vi "Argos_3.5 (K5 Customized Edition).vi"(0 "PID 1 COM":refnum<visa-resource-name>="COM1", 1 "START":bool, 2 "Write to File":bool, 3 "SP 1 input (°C)":dbl=20.0 min=0.0 max=1300.0, 4 "Intervall (s)":u32 max=600, 5 "Write/\nRead":bool=TRUE, 6 "Delay (ms)":u32=500 min=100 max=600000, 7 "Auto Tune":bool, 9 "Standby":bool, 11 "Reset\nSTOPP":bool, 12 "ON":bool=TRUE caption="OFF", 13 "Get Values":bool, 15 "File Path":path) -> (8 "(°C)":dbl format="%#.3f", 14 "SP 1 is (°C)":dbl)   [LabVIEW 2013]
doc: "1. Verwendung\n\nDas Programm dient der Steuerung und Abfrage des Thermocontrollers I3252 und dem Auslesen von zwei VC 840 Messgeräten und einem Druckmessgerät Pfeiffer Single Gauge. \nDie Messgeräte werden Standardmäßig ausgelesen und erst nach Betätigung des Schalters \"Write to File\" in einer Textdatei abgespeichert. Das Eingabefeld \"Intervall\" legt den Abstand der Messpunkte fest.\nDer Setpoint für den Thermocontroller wird erst nach Betätigung des Tasters \"Setpoint START\" übernommen und angesteuert. Er wird ind den EEPROM des Gerätes geschrieben. Die Regelung kann mit Hilfe des Schalters \"Standby\" unterbrochen werden. Durch den Taster \"Reset STOPP\" kann der Setpoint aus dem EEPROM gelöscht werden.\nDie Eingabeflächen \"Constant\" und \"Thickness\" dienen der Berechnung des spezifischen Widerstands.\nDie Eingabeflächen \"User\" und \"Sample\" werden in den Header der Textdatei übernommen.\nDer Indikator \"File Path\" zeigt den aktuellen Speicherort der Textdatei an. Dieser wird nach ausschalten des Schalters \"Write to File\" gelöscht. Bei erneuten Schreiben muss ein neuer Speicherort gewählt werden. Bei Wahl desselben Speicherorts werden sämtliche bereits gespeicherte Daten gelöscht.\n\n\n2. Erläuterungen zum Blockdiagramm\n2.1 äußere Sequenz\nDie äußerte Sequenz besteht aus fünf Frames. Der erste dient der Initialisierung der Ports. Der zweite dient als Verzögerung um dem Programm genug Zeit zu geben die Ports zu öffnen. Jedoch senden die beiden VC 840 bereits Informationen an den Computer die in einem Puffer zwischengespeichert werden. Im dritten Frame wird dieser Puffer geleert. Somit kommt es zu keinem Framing Error. Desweiteren wird in diesem Frame die Startzeit der Messungen genommen. Im vierten Frame wird die eigentliche Messung und Verarbeitung der Daten durchgeführt. Die while-Schleife wird nur durch Auftreten eines Fehlers oder durch Betätigung des Stopbuttons auf dem Front Panel in der oberen linken Ecke unterbrochen. Im fünften und letzten Frame werden die Ports wieder geschlossen und beim Auftreten eines Fehlers wird das Programm automatisch gestoppt. Falls kein Fehler auftritt wird die Sequenz von vorne abgearbeitet.\n\n2.2 while-Schleife und innere Sequenz\n2.2.1 \"Event Structure\"\n2.2.1.1 Allgemein\nDer erste Frame beinhaltet ein \"Event Structure\". Dieser reagiert auf insgesamt elf verschiedene Ereignisse. Falls keines dieser Ereignisse auftreten sollte, warte die Struktur eine Millisekunde bevor die \"Event Structure\" verlassen wird. Die übrigen Ereignisse treten ein, wenn der entsprechende Kontroller eine Werteänderung erfährt.\n\n2.2.1.2 Event: Setpoint\nDieser Case besteht von außen nach innen aus einer Stacked Sequence, einer for-Loop und einer Flat Sequence die wiederum zwei \"Case Structures\" enthält. Als erstes wird bei dem Schalter \"Setpoint START\" der Blinkmodus aktiviert und bei dem Schalter \"Read Temperature\" deaktiviert. Danach folgt das eigentliche setzen des Temperatursollwerts. In der ersten Iteration wird dem Controller I3252 ein Schreibbefehl gesendet. Theoretisch kann der Setpoint in den RAM oder in den EEPROM geschrieben werden. Diese Auswahl erfolgt mit Hilfe des Schalters \"RAM\". Da das Schreiben in den RAM -Speicher aber aus diversen Gründen nicht erwünscht ist, wurde es nicht implementiert. Eine nachträgliche Implementierung ist aber leicht möglich, in dem die untere String-Konstante \"*P012\" durch \"*W012\" ersetzt wird. An diesem Befehl wird eine fünfstellige Hexadezimalzahl angehängt, die den Sollwert wiedergibt. Der Sollwert wird vorher mit zehn multipliziert, da das Komma standardmäßig nach der ersten Ziffer festgesetzt wurde (Bsp.: 800 wird gesendet um 80 einzustellen). Dieser Befehlsstrang wird an das Gerät mittels des SubVIs \"Comm_Interface\", auf welches später noch näher eingegangen wird, weitergegeben. Der durch das Gerät zurückgegebene String wird nicht verarbeitet.\nDie zweite Iteration dient dem Auslesen des eingestellten Sollwertes. Wahlweise kann der RAM- oder der EEPROM-Speicher ausgelesen werden. Die eigentliche Verarbeitung des Ausgabestrings erfolgt durch das SubVI \"Edit Setpoint\".\nDie Implementierung zur Einstellung des zweiten Setpoints erfolgt durch kopieren der ersten beiden Fälle und ersetzen der \"1\" im Befehf durch eine \"2\" (Bsp.: \"*P012\" zu \"*P022\"). Es darf aber nicht vergessen werden, dass dann ebenfalls die Anzahl der Iterationen angepasst werden muss.\nAls letztes wird der Blinkmodus des Schalters \"Setpoint START\" wieder deaktiviert.\n\n2.2.1.3 Event: Standby\nDieses Ereignis aktiviert bzw. deaktiviert als erstes den Blinckmodus des entsprechenden Schalters und sendet danach den Befehl zum aktivieren (\"*D03\") oder zum deaktivieren (\"*E03\") des Standbymodus an den Thermocontroller.\n\n2.2.1.4 Event: Set Command \nDer in das Feld \"Command shall be\" eingegebene Befehl wird an den Thermocontroller übermittlet. Die korrekte Form des Befehls ist im \"Communication Manuel\" nachzuschlagen. Das \"*\"-Zeichen wurde allerdings schon implementiert und muss somit nicht mit eingegeben werden.\n\n2.2.1.5 Event: Reset\nIn der ersten Iteration wird der Reset-Befehl an den Thermocontroller gesendet. In Folge wird der gesamte EEPROM-Speicher gelöscht. Deshalb wird in der zweiten Iteration der Setpoint aktualisiert. Dieser Befehl hat keinen Einfluss auf den RAM-Speicher. Die anschließende Wartezeit ist auf vier Sekunden festgesetzt und wurde empirisch ermittelt. Diese Zeit benötigt das Gerät um den Reset durchzuführen und für die Kommunikation wieder zur Verfügung zu stehen.\n\n2.2.1.6 Event: Auto Tune\nEs ist festgeschrieben, dass der Setpoint für die \"Auto Tune\"-Funktion wenigstens 20°C über der aktuellen Temperatur liegt. Deshalb wird zunächst der aktuelle Temperaturwert ausgelesen. Im zweiten Schritt werden zu diesem Wert zwanzig addiert und der Setpoint wird in den RAM-Speicher geschrieben. Das Schreiben in diesen Speicher ist nötig, da die \"Auto Tune\"-Funktion\" erst nach einem Reset startet. Im dritten Schritt wird der eigentliche Befehl für den \"Auto Tune\" gesendet (siehe dazu \"Communication Manuel\" S.27). Als vierte und letzte Iteration der for-Schleife folgt der bereits erwähnte Reset-Befehl. Der Temperatursollwert, der im RAM-Speicher eingetragen ist, muss zum Schluss wieder auf 0°C gesetzt werden. Die Zeit für die Ausführung des \"Auto Tune\"-Befehls wurde empirisch ermittelt und 45 s festgesetzt.\n\n2.2.1.7 Event: Write LOW/HI\nDieses Ereignis setzt die am Analogausgang anliegende Spannung fest. Normalerweise beträgt dieser Spannungswert 0-10 V. Das angeschlossene Netzteil verträgt aber maximal nur 2,3 V. Aus diesem Grund wird der \"%HIGH\" auf 23 gesetzt. Somit beträgt die maximal anliegende Spannung nur noch 23% von der maximal möglichen, d.h 2,3V. Ein niedrigerer Wert ist jederzeit möglich, genauso wie ein höherer für den Parameter \"%LOW\". Diese werden zunächst nacheinander in den RAM-Speicher geschrieben und anschließend wieder ausgelesen.\n\n2.2.1.8 Event: Set PID\nDie Werte für den PID-Regler können sowohl mit Hilfe der \"Auto Tune\"-Funktion, als auch manuell eingestellt werden. Es wird wiederum zwischen dem Schreiben in den RAM- und dem EEPROM-Speicher unterschieden. Zunächst werden die Werte für \"P\", \"I\" und \"D\", in dieser Reihenfolge, gesetzt und danach die aktuellen Werte ausgelesen.\n\n2.2.1.9 Event: Get Values\nDieses Ereignis hat zur Folge, dass die Werte für \"P\", \"I\", \"D\", \"%LOW\", \"%HIGH\" und des Setpoints wahlweise aus dem RAM- oder EEPROM-Speicher gelesen werden. Die aktuellen Werte werden nicht nur in die entsprechenden Anzeigefelder übernommen, sondern auch in die entsprechenden Eingabefelder, mit Ausnahme des Temperatursollwerts. \n\n2.2.1.10 Event: RAM\nPrinzipiell kann zwischen dem Schreiben in den RAM- oder EEPROM-Speicher des Thermocontrollers gewählt werden. Die entsprechende Schalterposition auf dem Frontpanel zeigt den aktuell verwendeten Speicher an. Die Anzeigewerte werden bei jedem Umschalten aktualisiert und sind im entsprechenden Speicher eingetragen. Die Implementierung ist identisch mit der des Ereignisses \"Get Values\". Es gilt zu beachten, dass die Werte für \"%LOW\" und \"%HIGH\" nur in den RAM-Speicher geschrieben werden können und somit auch nur aus diesem ausgelesen werden können.\n\n2.2.1.11 Event: Set Gauge to Zero\nMit Hilfe der SubVIs \"Get Pressure\" und \"Offset Display\" werden die Werte für den alten und den neuen Offset und der durch den zweiten Drucksensor ermittelt Druck ermittelt. \n\n2.2.1.12 Event: Write to File\nSollte der Schalter \"Write to File\" aktiviert werden, d.h. Schalterposition oben, so wird zunächst durch das SubVI \"Header\" ein Header für die unter \"File Path\" definierte Datei angelegt. Alle Werte, die bereits in der entsprechenden Datei stehen, werden dabei gelöscht.\n\n2.2.2 \"Timed Structures\"\nIm dritten Frame der inneren Sequenz werden die Werte für Zeitpunkt, Temperatur, Spannung, Strom und Druck ermittelt. Damit die Werte zum gleichen Zeitpunkt aufgenommen werden, werden \"Timed Sequences\" eingesetzt. Mit dem entsprechenden Schalter auf dem Front Panel unter dem Tab \"Settings\" kann gewählt werden, ob das entsprechende Gerät ausgelesen werden soll oder nicht. Die einzelnen Sequenzen werden parallel abgearbeitet, womit die Prozesszeit von diesem Frame durch der zeitintensivsten Sequenz abhängt. Dies ist in aller Regel das Auslesen der Temperatur, da ein \"Delay\" von 500 ms oder größer benötigt wird, um den Controller ordentlich ansprechen zu können.\nDie Systemzeit wird durch das SubVI \"System Time in Seconds\" in Sekunden umgerechnet und der in dem Parameter \"Starttime\" gespeicherte Wert wird abgezogen. Somit werden die Sekunden seit dem Start des Programms gezählt.\n\n2.2.3 restlichen Frames\nIm zweiten Frame wird das Intervall zwischen den einzelnen Messwerten festgelegt. Dabei wird der Wert des Parameters \"Delay\" abgezogen. Dieser Wert beträgt im Normalfall 500 ms und ist somit nicht vernachlääsigbar.\nDer Vierte Frame beinhaltet die Umrechnung des Temperatur-Strings in einen Temperaturwert durch das SubVI \"Edit Tmperature\", die Berechnung des spezifischen Widerstands durch das SubVI \"Resistivity Calculation\" und die Überprüfung des Druckwerts. Auch werden die neu gewonnen Werte in das entsprechende Shift-Register übernommen. Falls der Druckwert einen in dem Parameter \"Pressure Limit (mbar)\" festgelegten Grenzwert überschreiten sollte, wird der Thermocontroller automatisch in den Standby-Modus versetzt. Des Weiteren wird der Schalter \"Standby\" solange gesperrt, wie der Druck oberhalb des Grenzwertes liegt. Wenn der Druck wieder unter den Grenzwert gesunken ist, wird der Standby-Befehl nicht automatisch aufgehoben, sondern muss vom Benutzer durch Betätigung des entsprechenden Schalters gegeben werden.\nIm fünften Frame werden die Diagramme erstellt. Dabei wird jedes Mal von neuem das gesamte Shift-Register als Graph dargestellt. Weiterhin werden die Messwerte in ein 1D-Array geschrieben.\nDer sechste und letzte Frame beinhaltet den eigentlich Schreibvorgang der Messwerte in eine Textdatei und die Überprüfung ob ein Fehler vorliegt.\n\n2.3 SubVIs\n2.3.1 Allgemein\nDie SubVIs für die Messgeräte VC840 und das Druckmessgerät wurden aus anderen Quellen übernommen. \n\n2.3.2 \"Header\"\nIn den Header wird zunächst das aktuelle Datum und die aktuelle Zeit übernommen. Die ausgewählte Datei wird dabei überschrieben. Danach wird der Name des Benutzers und der Probe übernommen. Zum Schluss werden die Einheiten in einer Reihe, durch einen Tabulator getrennt, in den Header geschrieben.\n\n2.3.3 \"I3252 Comm Interface\"\nDieses VI stellt die Kommunikation mit dem Thermocontroller her und gibt den Ausgabe-String zurück.\n\n2.3.4 \"I3252 Edit Setpoint\"\nIm Ausgabe-String vom Thermocontroller ist an der vierten Stelle die Stelle des Dezimalpunktes verschlüsselt. Dieses Hexadezimalzahl wird herausgefiltert und an ein \"ENUM Controller\" übergeben. Dieser weist der Hexadezimalzahl eine Nummer zu, mit welcher ein Wert aus einem Array entnommen wird. Dieser Wert dient als Quotient. Der tatsächliche Wert kann somit errechnet werden.\n\n2.3.5 \"I3252 Edit Temperature\"\nDer Temperatur-String, der vom Thermocontroller zurückgegeben wird, wird in eine Dezimalzahl umgewandelt. Manchmal kommt es aus zu Dropouts, die durch dieses Programm herausgefiltert werden. Der letzte Wert wird dabei in einer \"Feedback Node\" gehalten unter der Annahme, dass sich der Temperaturwert nicht sprunghaft ändert.\n\n2.3.6 \"Resistivity Calculation\"\nDer spezifische Widerstand wird nach folgender Formel ausgerechnet. Dabei entspricht t der Dicke der Probe und C ist eine Konstante.\nrho=C*pi*t*U/(ln( 2)*I)\n\n2.3.7 \"System Time in Seconds\"\nZunächst wird die aktuelle Systemzeit ausgelesen. Danach wird diese in Stunden, Minuten und Sekunden aufgeteilt, alles in Sekunden umgerechnet und letztendlich addiert."
uses:
  <vilib>/Platform/TimedLoop/XDataNode/timing_clust.ctl
  <vilib>/Platform/TimedLoop/XDataNode/nitl_modes.ctl
  <vilib>/Platform/TimedLoop/XDataNode/wakeup.ctl
  <vilib>/Instr/_visa.llb/VISA Configure Serial Port (Instr).vi
  <vilib>/Platform/TimedLoop/scheduler/LVUserAPI/_suppVIs/Create_1kHz_TSource.vi
  <vilib>/Utility/file.llb/Write To Spreadsheet File (DBL).vi
  <vilib>/Platform/TimedLoop/XDataNode/XDataNode.xnode
  <vilib>/Platform/TimedLoop/XDataNode/XDNodeRunTimeDep.lvlib
  D:/Argos_K_1.99 (SUPTNIK Customized Edition)/Dependencies/Pfeiffer TPG261+262 Single+Dual Gauge/Dual Gauge.lvlib
panel:
  out "Resistivity/ Temp Dependency":cluster{dbl[], dbl[]}(graph)
  out "read buffer":string
  out "appended array":dbl[](array[numeric])
  in  "Tab Control":T1(tab)
  in  "Soak time (min)":dbl
  in  "Ramp time (min)":dbl
  in  "RAMP":bool
  in  "Set Value":bool
  in  "OUTPUT":bool
  in  "4PP Const":dbl=1.0
  in  "Thickness":dbl=40.0
  in  "Voltage\nCompl.":dbl=2.0
  in  "Unit   2":string(combo)="0"
  in  "Unit":string(combo)="1"
  in  "Source \nCurrent":dbl=20.0
  in  "Sample":string
  in  "User":string
  out "Thermocouple":cluster{dbl[], dbl[]}(graph)
  out "current time (s)":dbl
  out "data logger intervall (s)":dbl
  out "loop time (s)":dbl
  in  "stop":bool
  out "TPG 1":cluster{dbl[], dbl[]}(graph)
  out "Pressure Baratron 2":dbl format="%#_4e"
  out "Resistivity Graph":cluster{dbl[], dbl[]}(graph)
  out "Resistivity\n 2":dbl
  out "Voltage Graph":cluster{dbl[], dbl[]}(graph)
  out "Current Graph":cluster{dbl[], dbl[]}(graph)
  out "Voltage\n 2":string
  out "Current \n3":string
  in  "Keithley Port":refnum<visa-resource-name>="COM6"
  out "status 2":bool caption="Status"
  out "code 2":i32 caption="Code"
  out "code":i32 caption="Code"
  out "status":bool caption="Status"
  in  "Set Gauge to Zero":bool
  out "Status Gauge 1#2":i32(ring) items=["data OK", "underrange", "overrange", "sensor error", "sensor off", "no sensor", "ID error"]
  out "Pressure Gauge 1#2":dbl format="%.3e"
  out "Pressure Gauge 1#1":dbl format="%.3e"
  out "Status Gauge 1#1":i32(ring) items=["data OK", "underrange", "overrange", "sensor error", "sensor off", "no sensor", "ID error"]
  in  "TPG 1 COM":refnum<visa-resource-name>="COM5"
  in  "Pressure Limit (mbar)":dbl=1.0 min=0.0 max=1100.0
  out "Current Offset (mbar)":dbl
  in  "ON (TPG 2)":bool caption="OFF"
  in  "ON (TPG 1)":bool=TRUE caption="OFF"
  in  "ON":bool caption="OFF"
  in  "VC 840 2":refnum<visa-resource-name>="COM4"
  out "Reading 2":dbl format="%_4f"
  out "Mode 2":enum16{"?", "Diode", "Beep", "DC", "AC"}(ring)
  out "Unit 2":string
  in  "VC 840 1":refnum<visa-resource-name>="COM4"
  out "Reading 1":dbl format="%_4f"
  out "Mode 1":enum16{"?", "Diode", "Beep", "DC", "AC"}(ring)
  out "Unit 1":string
  out "Status 1":T2
  out "Status 2":T2
  in  "ON":bool caption="OFF"
  out "% HIGH Istwert":u32
  out "% LOW Istwert":u32
  in  "% High Sollwert":u32=23 max=24
  in  "% LOW Sollwert":u32 max=25
  in  "RAM":bool=TRUE caption="EEPROM"
  out "D (Rate) IstWert":u32
  out "I ( Reset1) Istwert":u32
  out "P (PB1) Istwert":u32 caption="actual value"
  in  "D (Rate) Sollwert":u32 max=3999
  in  "I ( Reset1) Sollwert":u32 max=3999
  in  "P (PB1) Sollwert":u32 caption="set value" max=9999
  in  "Set Command":bool
  in  "Set PID":bool
  in  "Write LOW/HI":bool
  in  "Flow Control":u16(ring) items=["None"=0, "XON/XOFF"=1, "RTS/CTS"=2, "DTR/DSR"=4]
  in  "Stop Bits":u16(ring)=10 items=["1.0"=10, "1.5"=15, "2.0"=20]
  in  "Parity":u16(ring)=1 items=["None", "Odd", "Even", "Mark", "Space"]
  in  "Data Bits":u16=7 min=5 max=8 step=1
  in  "Baud Rate":u32=9600
  out "Command output":string
  in  "Command input":string
  in  "TPG 2 COM":refnum<visa-resource-name>="COM4"
  out "Pressure Gauge 2#2":dbl format="%.3e"
  out "Pressure Gauge 2#1":dbl format="%.3e"
  out "Status Gauge 2#2":i32(ring) items=["data OK", "underrange", "overrange", "sensor error", "sensor off", "no sensor", "ID error"]
  out "Status Gauge 2#1":i32(ring) items=["data OK", "underrange", "overrange", "sensor error", "sensor off", "no sensor", "ID error"]
  out "Pirani (VVP1 Scroll)":cluster{dbl[], dbl[]}(graph)
  in  "4PP constant":dbl min=0.0 max=5.0
  in  "Thickness (nm)":dbl min=0.0
  out "Pressure Pirani 2":dbl format="%#_3e"
  in  "Minutes":dbl
  in  "Hours":dbl
  in  "Soak Minutes":dbl=1.0
  in  "Soak Hours":dbl
  out "Actual SetPoint":dbl
  in  "Get SetPoint":bool
  # "set \nvalue"
  # "actual \nvalue"
  # "T (°C)"
  # "nm"
  # "Ohm Cm"
  # "mbar"
  # "Amps"
  # "Pressure Measurement \n(Pfeiffer TPG261)"
  # "PID Controller (Omega Newport i3252)"
  # "Keithley 4PP measurement"
  # "Ramp And Soak Toolkit"
  # "limit (mbar)"
  # "Multimeter\n#1 (VC 840)"
  # "Multimeter\n#2 (VC 840)"
  # "P"
  # "I"
  # "D"
  # "% Low"
  # "% High"
  # "mbar"
  # "Ramp"
  # "Soak"
  # "Authors:  Daniel Schuster (sir-dan@web.de)\n                 Steffen Cornelius (s.cornelius@hzdr.de)\n                 Nico Spahn (x)\n\n                 premade SubVIs for readout of Pfeiffer gauge and VC840 Multimeters were used\n                 SubVI \"I3252_Comm_Interface\" is based on a modified Labview example\n\nRelease:  v1.0    \n\nVersion History:\n\nv1.1  -    28.06.2011\n             - Format des Files geändert von %.3f auf %g\n             - maximale Eingabewerte für PID begrenzt\nv1.2  -    12.07.2011\n             - Anzeige p,rho, U, V auf Scientific geändert\n             - y-Achse p,rho auf Log geändert\n             - numerische Zeitanzeige hinzugefügt\n             - 4PP Constant: pi/ln(2)=4,532 set as the default value\nv1.3  -    25.07.2011\n             - Zeitvariable auf EXT geändert, um Sprünge in Diagrammen loszuwerden\nv1.4  -   27.07.2011\n             - ALLE Variablen auf DBL zurückgesetzt wegen Formatierungsproblem im File\n             - Zeitberechnung neu gemacht (Tick count differenzen) -> Zeitsprünge korrigiert ?\n             - Delay/Intervall überarbeitet\nv1.5  -   05.12.2012\n                - Austausch der alten Pfeifer SubvIs durch neue -> nun alle 4 Kanäle des DualGauge\n                                                                                                         Controllers gleichzeitig auslesbar\n                - neue Pfeiffer SubVIs verwendet in Druckwertauslesung und Offset Berechnung des Baratron\n                  Druckes (COM5 Sensor1)\n                - Neuarragement des GUI -> FullRange und Baratron neben Temperatur auf Haupseite zu sehen\n                                                                   Pirani und OpenPort auf Meas.2 zu sehen\n                                                                   Diagnose Seite umfasst nun auch Widerstandsdiagramm\n                - Änderungen der Settingseite -> nun alle 4 Drucksensoren mit aktuellem Messwert und Gerätestatus\n                                                                           zu sehen\n                - The readout of the PID-Temperature Controller and the VC840 Multimeters was not modified\nv1.73  -  18.10.2013\n                - Layout Änderungen\nv.1.8   -  19.01.2014\n                - Änderung Layout Settings Tab\n                - Trennung der beiden TPG Dual Gauge Controls\n                -"
  # "Version 1.73    - last change 18.10.2013"
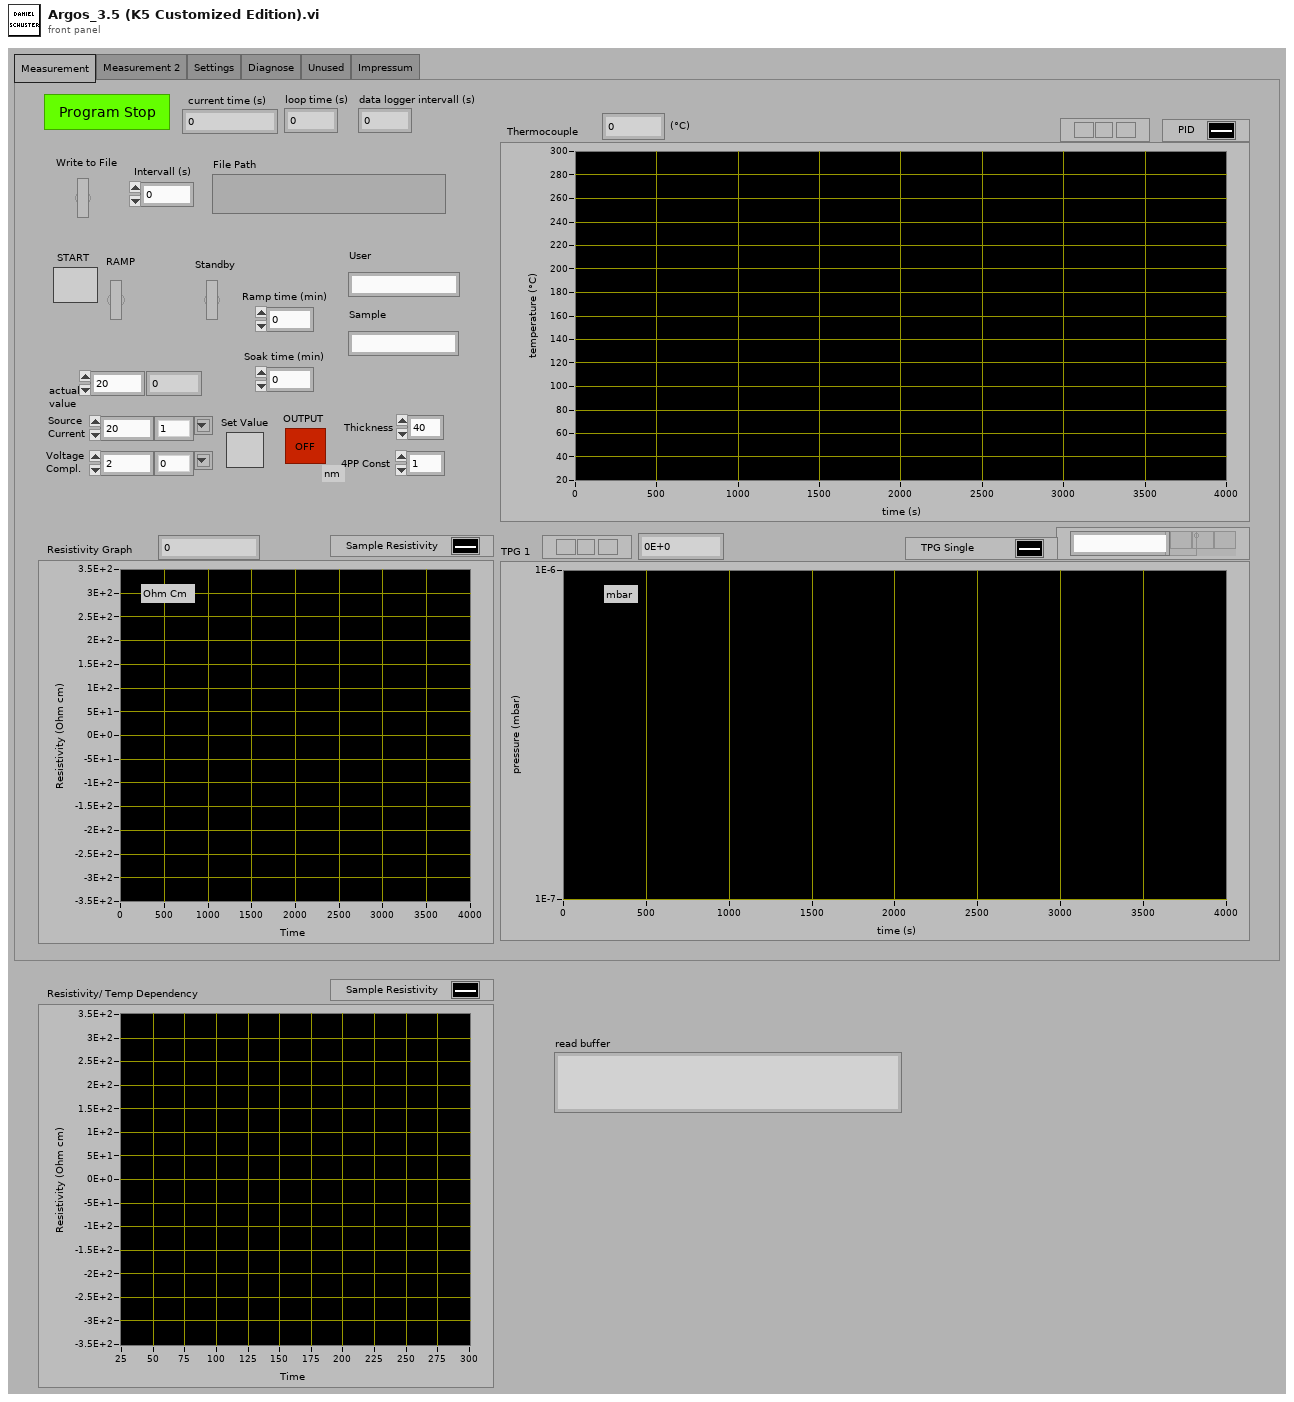
[diagram p1: front panel]
types:
  T1 = enum32{"Measurement", "Measurement 2", "Settings", "Diagnose", "Unused", "Impressum"}
  T2 = cluster{"Low Bat":bool, "Auto":bool, "Delta":bool, "Hold":bool, "RS232":bool}
  T3 = typedef "XDNodeRunTimeDep.lvlib/timing_clust.ctl" = cluster{"Expected End [f-1]":u64, "Actual End [f-1]":u64, "Finished Late? [f-1]":bool, "Expected End [i-1]":u64, "Actual End [i-1]":u64, "Finished Late? [i-1]":bool, "Expected Start [i]":u64, "Actual Start [i]":u64, "Expected Start [f]":u64, "Actual Start [f]":u64, "Source Name":string, "Structure Name":string, "Period":i64, "Deadline":i64, "Offset":i64, "Start":i64, "Priority":i32, "Timeout":i32, "Mode":T4, "Wakeup Reason":T5, "Error":errorcluster, "Source Type":string, "Secondary Source Type":string, "Global End Time":u64, "Global Start Time":u64, "Frame Duration":u64, "Iteration Duration":u64, "Assigned CPU":i32, "I/O Scan Engine Mode":u32}
  T4 = typedef "XDNodeRunTimeDep.lvlib/nitl_modes.ctl" = enum32{"No Change", "Process missed periods, maintain original phase", "Discard missed periods, maintain original phase", "Process missed periods, ignore original phase", "Discard missed periods, ignore original phase"}
  T5 = typedef "XDNodeRunTimeDep.lvlib/wakeup.ctl" = enum32{"Normal", "Aborted", "Asynchronous wakeup", "Timing source error", "Timed loop error", "Timeout"}
  T6 = enum8{"Enabled", "Disabled", "Disabled and Grayed Out"}
  T7 = cluster{"VISA resource name out":refnum<visa-resource-name>, "error out":errorcluster, "Delay (ms)":u32, "Write/\nRead":bool}
  T8 = cluster{"TPG 2 COM":refnum<visa-resource-name>, "error out":errorcluster}
  T9 = cluster{"COM out":refnum<visa-resource-name>, "Cluster (Ausgang)":errorcluster}
  T10 = cluster{"Pressure Gauge#1":dbl, "Pressure Gauge#2":dbl}
  T11 = cluster{"TPG 1 COM":refnum<visa-resource-name>, "error out":errorcluster}
  T12 = cluster{"COM out":refnum<visa-resource-name>, "error out":errorcluster, "COM out":refnum<visa-resource-name>, "error out":errorcluster}
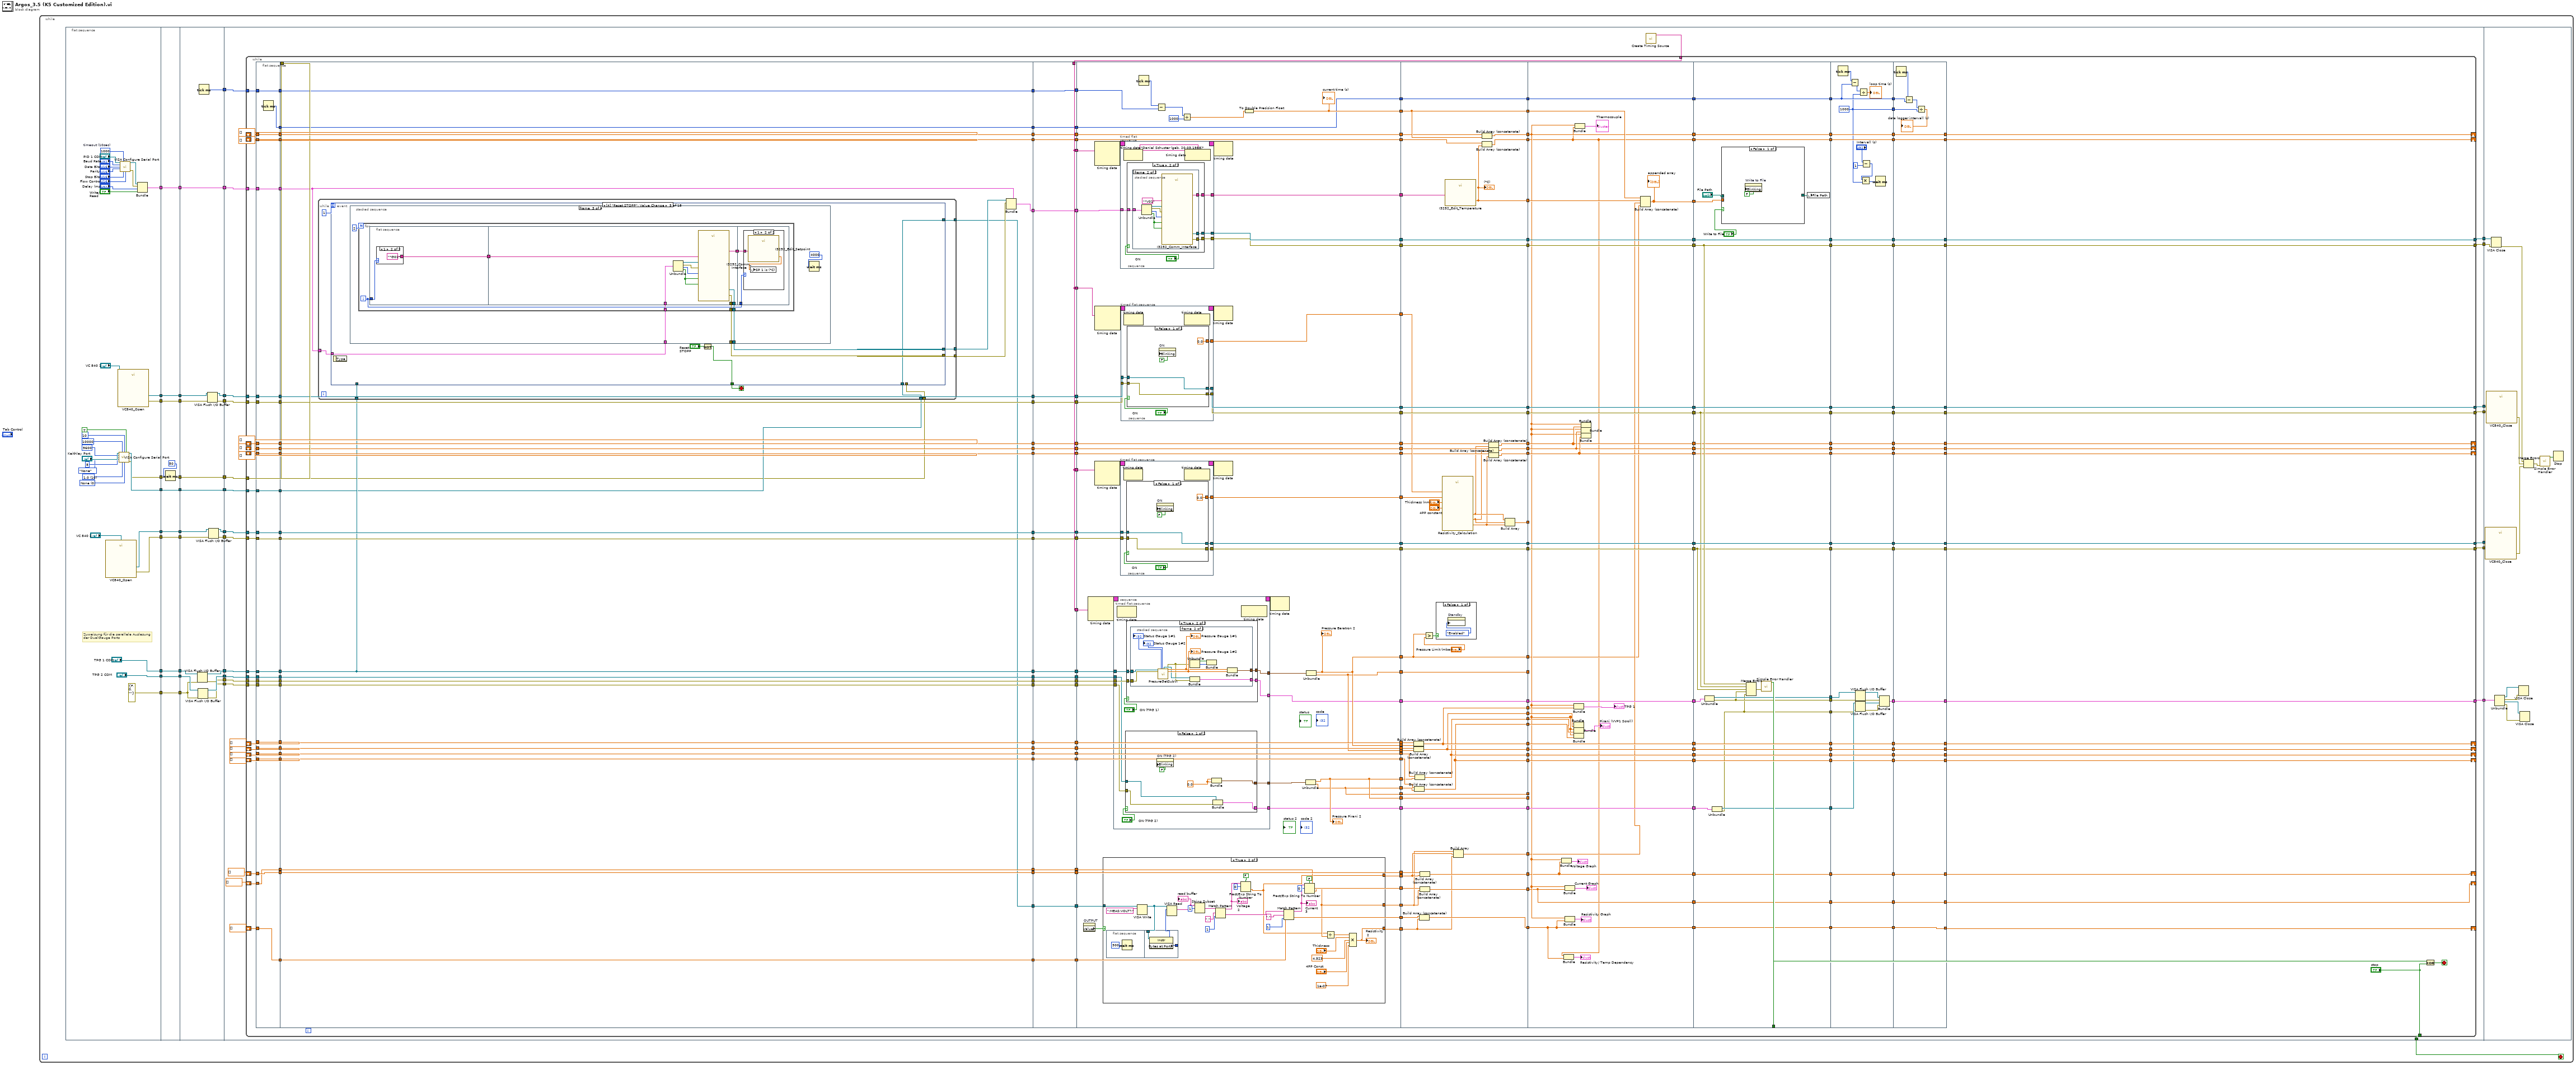
[diagram p0: block diagram]
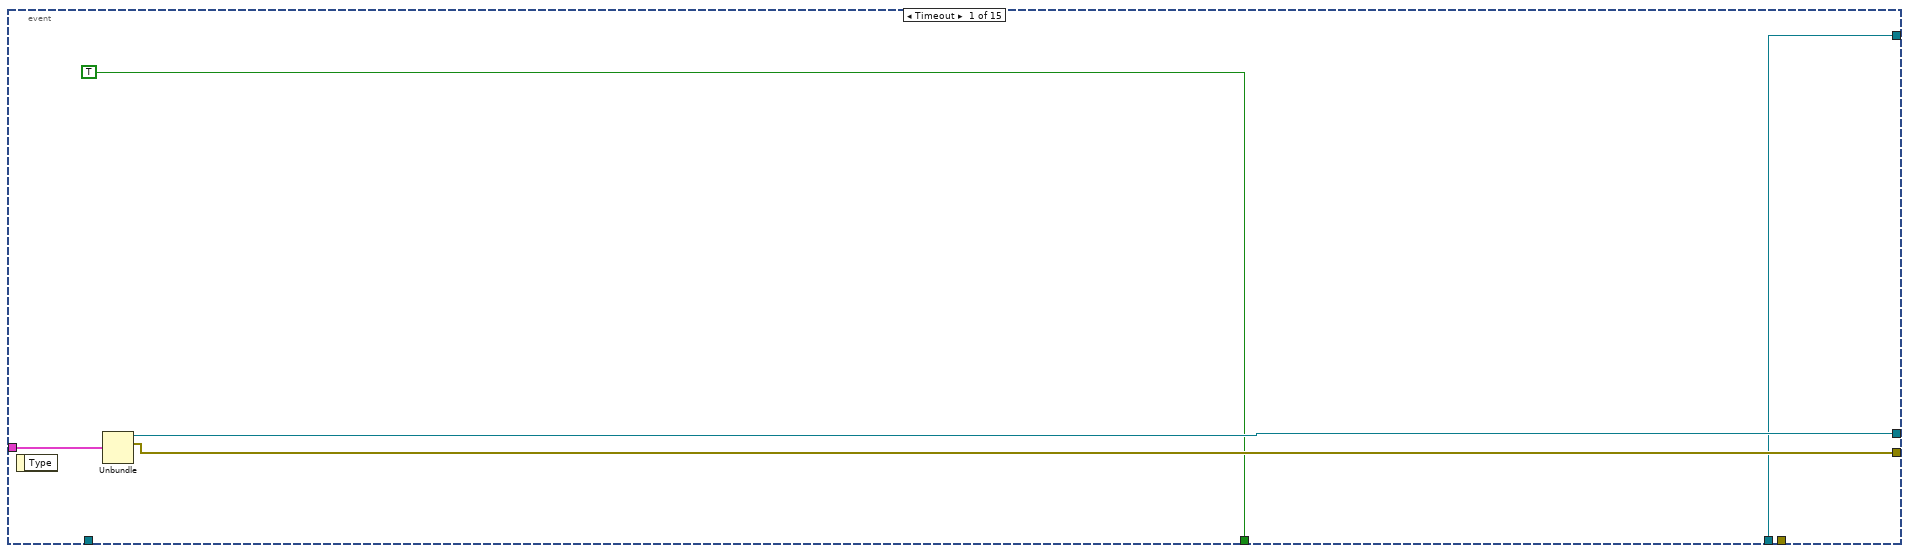
[diagram p2: hidden frame]
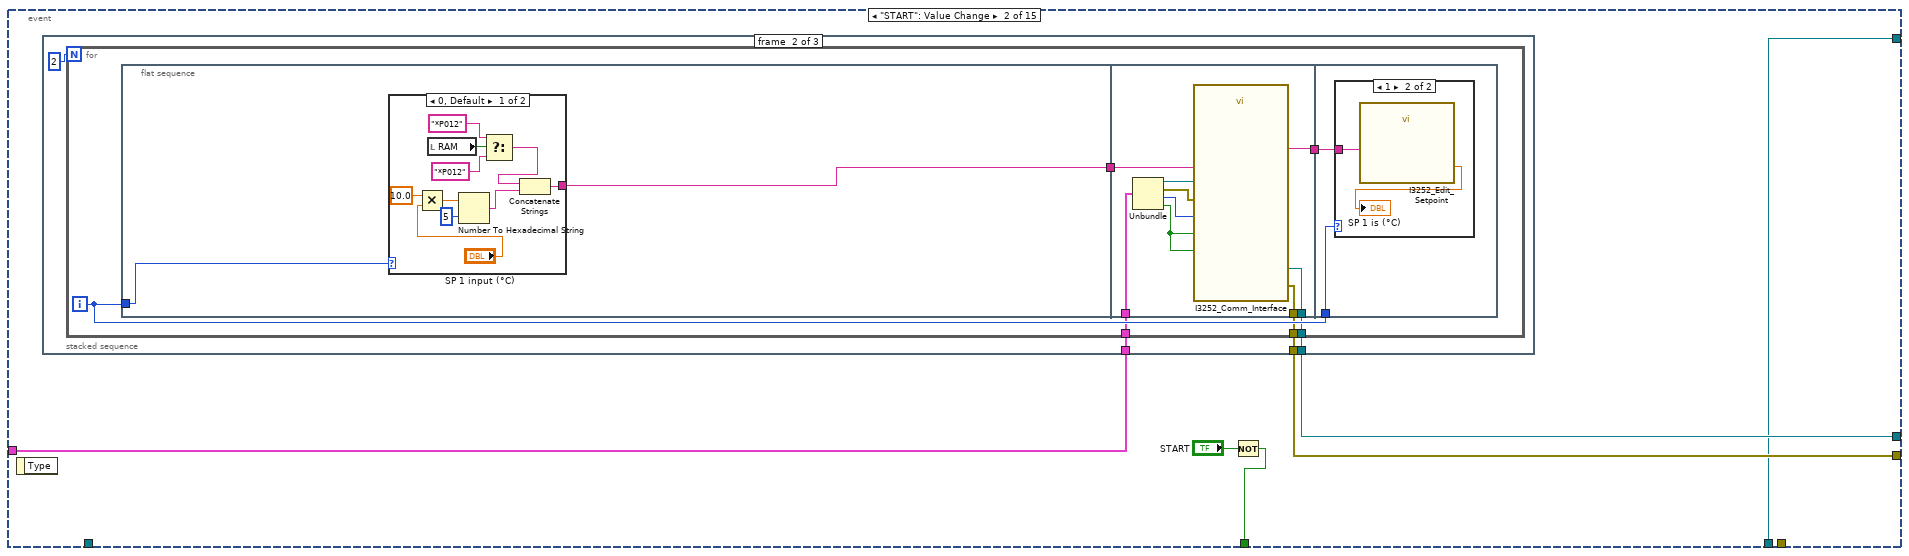
[diagram p3: hidden frame]
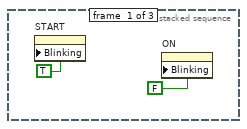
[diagram p4: hidden frame]
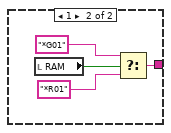
[diagram p5: hidden frame]
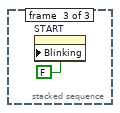
[diagram p7: hidden frame]
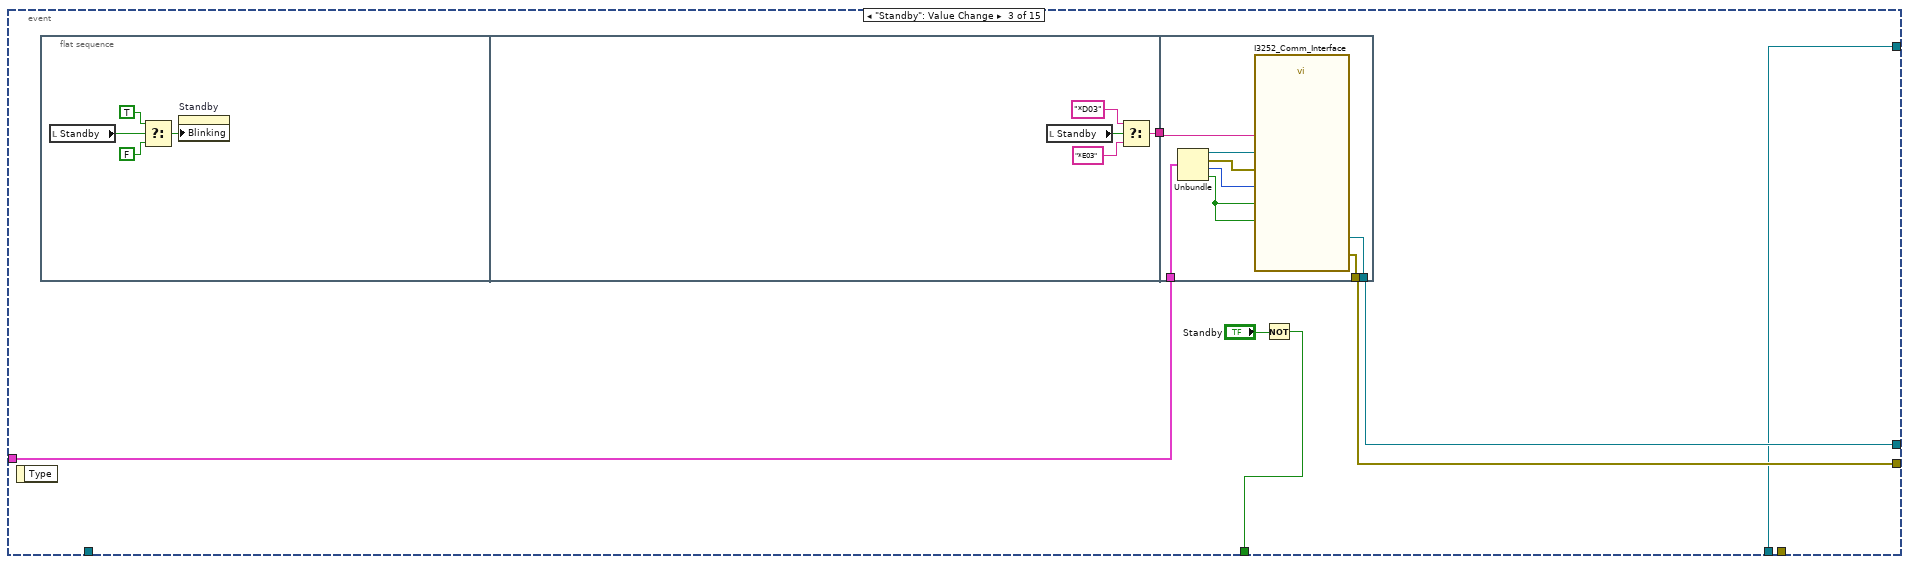
[diagram p8: hidden frame]
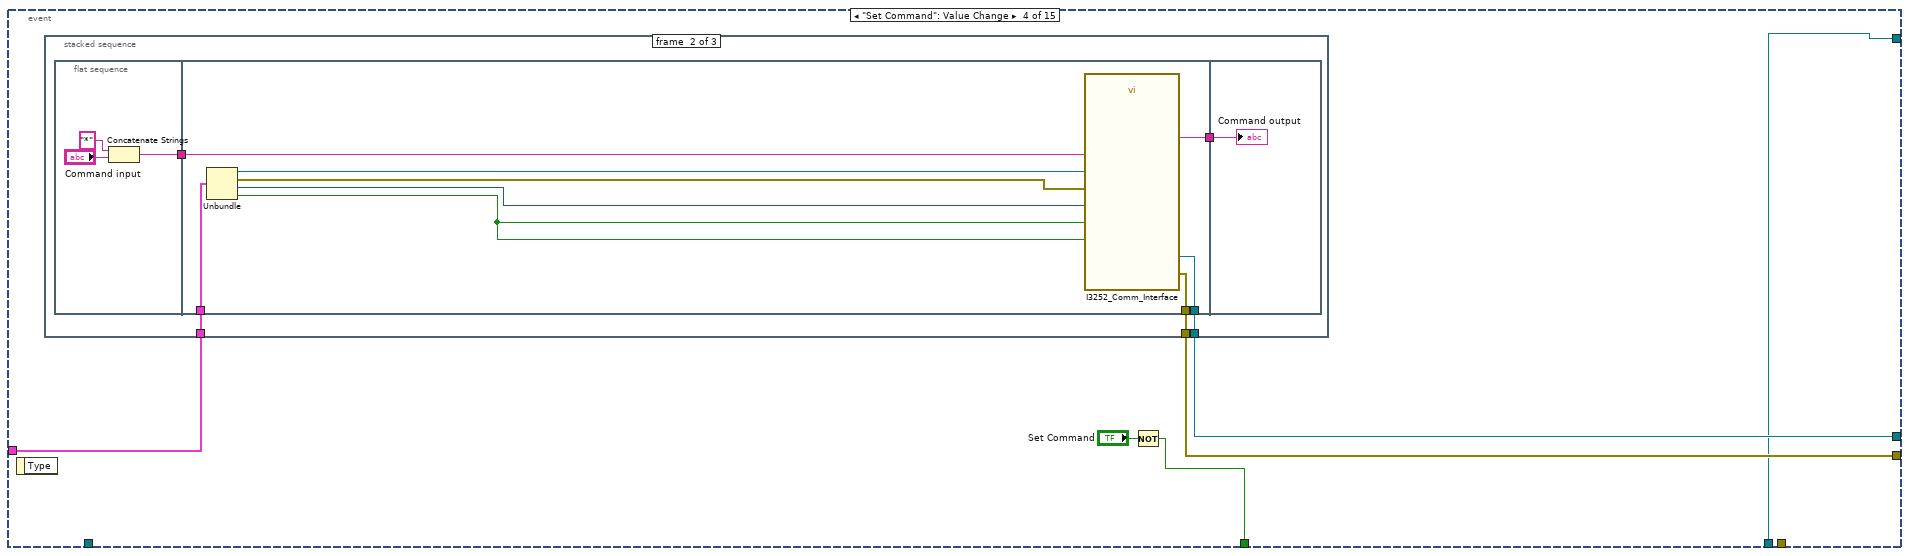
[diagram p9: hidden frame]
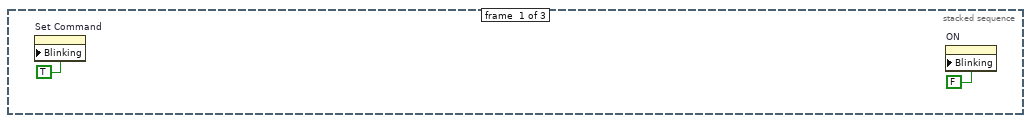
[diagram p10: hidden frame]
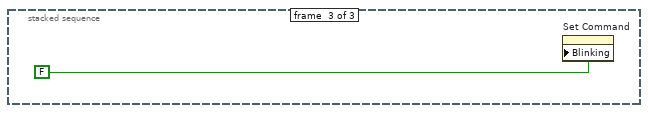
[diagram p11: hidden frame]
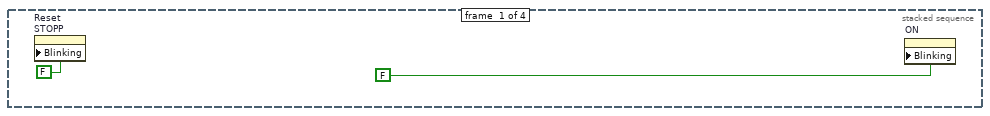
[diagram p12: hidden frame]
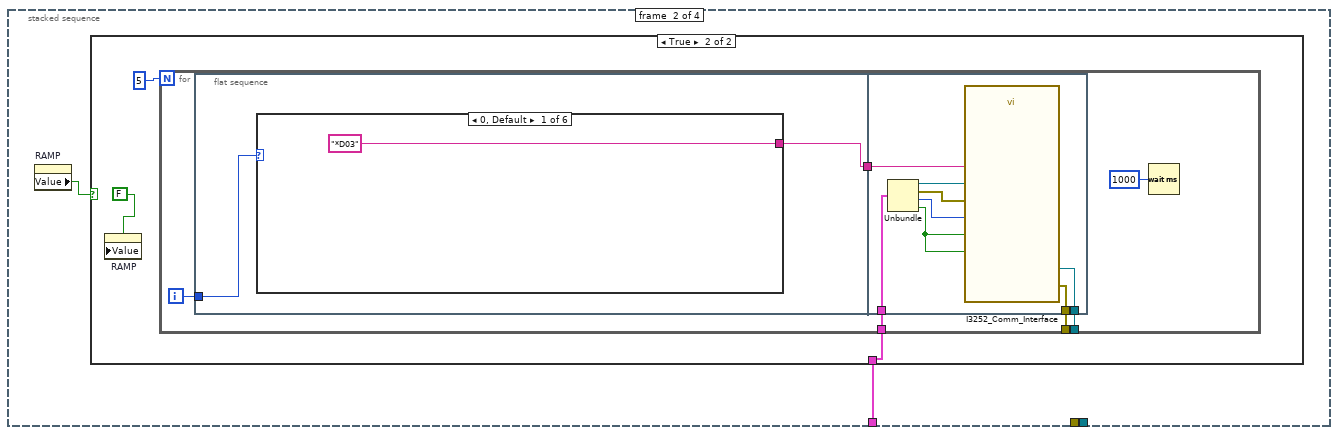
[diagram p13: hidden frame]
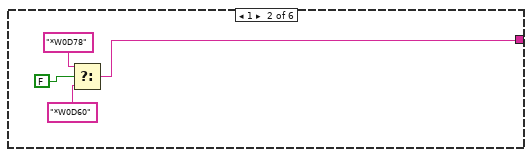
[diagram p15: hidden frame]
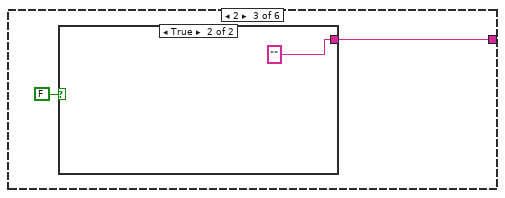
[diagram p16: hidden frame]
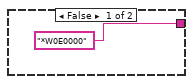
[diagram p17: hidden frame]
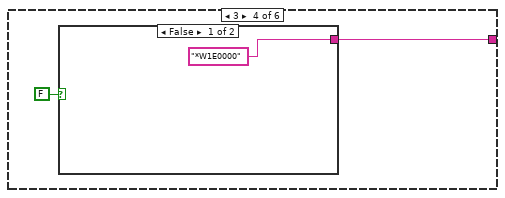
[diagram p18: hidden frame]
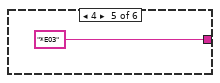
[diagram p20: hidden frame]
diagram:
  n1 = while {
    stop <- w12 stop-if-true
    n2 = flat-sequence {
      tunnel: [w71] -> w40
      tunnel: [w72] -> w39
      tunnel: [w57] -> w38
      tunnel: [w70] -> w37
      tunnel: [w69] -> w36
      tunnel: ["TPG 1 COM"] -> w35
      tunnel: ["TPG 2 COM"] -> w34
      tunnel: [errorcluster {"status"=FALSE, "code"=0, "source"=""} ("Fehler (Eingang)")] -> w9
      tunnel: [w42] -> w4
      tunnel: [w41] -> w3
      tunnel: w40 -> [w83]
      tunnel: [w83] -> w33
      tunnel: w39 -> [w82]
      tunnel: [w82] -> w32
      tunnel: w38 -> [w81]
      tunnel: [w81] -> w31
      tunnel: w37 -> [w80]
      tunnel: [w80] -> w30
      tunnel: w36 -> [w79]
      tunnel: [w79] -> w29
      tunnel: [w77] -> w28
      tunnel: w35 -> [w77]
      tunnel: [w76] -> w27
      tunnel: w34 -> [w76]
      tunnel: [w75] -> w10
      tunnel: w9 -> [w75]
      tunnel: [w74] -> w5
      tunnel: w4 -> [w74]
      tunnel: w3 -> [w73]
      tunnel: [w73] -> w2
      tunnel: w33 -> [w96]
      tunnel: [w95] -> w26
      tunnel: w32 -> [w97]
      tunnel: [w94] -> w25
      tunnel: w31 -> [w102]
      tunnel: [w102] -> w24
      tunnel: w30 -> [w99]
      tunnel: [w100] -> w23
      tunnel: w29 -> [w98]
      tunnel: [w101] -> w22
      tunnel: [w93] -> w21
      tunnel: [w91] -> w20
      tunnel: w28 -> [w92]
      tunnel: [w90] -> w19
      tunnel: w27 -> [w89]
      tunnel: w10 -> [w88]
      tunnel: [w87] -> w8
      tunnel: [w86] -> w7
      tunnel: [w85] -> w6
      tunnel: w5 -> [w85]
      tunnel: w2 -> [w84]
      tunnel: [w84] -> w1
      tunnel: w26 -> [w135]
      tunnel: w25 -> [w134]
      tunnel: w24 -> [w133]
      tunnel: w23 -> [w131]
      tunnel: w22 -> [w130]
      tunnel: [w129] -> w18
      tunnel: [w128] -> w17
      tunnel: [w127] -> w16
      tunnel: [w126] -> w15
      tunnel: [w125] -> w14
      tunnel: [w124] -> w13
      tunnel: w21 -> [w118]
      tunnel: w20 -> [w117]
      tunnel: w19 -> [w116]
      tunnel: [w111] -> w12
      tunnel: [w110] -> w11
      tunnel: w8 -> [w109]
      tunnel: w7 -> [w108]
      tunnel: w6 -> [w107]
      tunnel: w1 -> [w106]
      tunnel: w18 -> [w1640]
      tunnel: w17 -> [w1639]
      tunnel: w16 -> [w1642]
      tunnel: w15 -> [w1641]
      tunnel: w14 -> [w1644]
      tunnel: w13 -> [w1643]
      tunnel: w11 -> [w1637]
      frame #0 {
        w43 = u16 0 items=["None", "XON/XOFF", "RTS/CTS", "XON/XOFF & RTS/CTS", "DTR/DSR", "XON/XOFF & DTR/DSR"] ("flow control (0:none)")
        w44 = u16 10 items=["1.0"=10, "1.5"=15, "2.0"=20] ("stop bits (10: 1 bit)")
        w58 = u32 1000  # timeout (10sec)
        # "Zuweisung für die parallele Auslesung\nder DualGauge Ports"
        n3 = call "VC840_Open.vi"("VISA resource name"="VC 840 2") -> ("error out"=w69:errorcluster, "VISA resource name out"=w70:refnum<visa-resource-name>)  [unwired: 1 in, 8 out]
        n4 = call "VC840_Open.vi"("VISA resource name"="VC 840 1") -> ("error out"=w72:errorcluster, "VISA resource name out"=w71:refnum<visa-resource-name>)  [unwired: 1 in, 8 out]
        n5 = call-poly "VISA Configure Serial Port"("VISA resource name"="Keithley Port", "timeout (10sec)"=u32 10000, "termination char\n(0xA = '\\n' = LF)"=u8 10 ("termination char\n(0xA = '\\n' = LF)"), "Enable Termination\nChar (T)"=TRUE ("Enable Termination\nChar (T)"), "baud rate (9600)"=u32 9600, "data bits (8)"=u16 8, "parity (0:none)"=enum16{"None", "Odd", "Even", "Mark", "Space"}."None", "stop bits (10: 1 bit)"=w44, "flow control (0:none)"=w43) -> ("VISA resource name out"=w42:refnum<visa-resource-name>, "error out"=w41:errorcluster)  [unwired: 5 in]
        n6 = call-poly "VISA Configure Serial Port"("VISA resource name"="PID 1 COM", "timeout (10sec)"=w58, "baud rate (9600)"="Baud Rate", "data bits (8)"="Data Bits", "parity (0:none)"="Parity", "stop bits (10: 1 bit)"="Stop Bits", "flow control (0:none)"="Flow Control") -> ("VISA resource name out"=w67:refnum<visa-resource-name>, "error out"=w68:errorcluster)  [unwired: 2 in, 5 out]
        n7 = Bundle("VISA resource name out"=w67, "error out"=w68, "Delay (ms)"="Delay (ms)", "Write/\nRead"="Write/\nRead") -> (w57:T7)  [unwired: 1 in]
      }
      frame #1 {
        n8 = Wait (ms)(milliseconds to wait=u32 50) -> ()  [unwired: 1 out]
      }
      frame #2 {
        n9 = VISA Flush I/O Buffer(VISA resource name=w92, error in (no error)=w88) -> (VISA resource name out=w91:refnum<visa-resource-name>, error out=w87:errorcluster)  [unwired: 1 in]
        n10 = VISA Flush I/O Buffer(VISA resource name=w89, error in (no error)=w88) -> (VISA resource name out=w90:refnum<visa-resource-name>, error out=w86:errorcluster)  [unwired: 1 in]
        n11 = Tick Count (ms)() -> (millisecond timer value=w93:u32)
        n12 = VISA Flush I/O Buffer(VISA resource name=w96, error in (no error)=w97) -> (VISA resource name out=w95:refnum<visa-resource-name>, error out=w94:errorcluster)  [unwired: 1 in]
        n13 = VISA Flush I/O Buffer(VISA resource name=w99, error in (no error)=w98) -> (VISA resource name out=w100:refnum<visa-resource-name>, error out=w101:errorcluster)  [unwired: 1 in]
      }
      frame #3 {
        n14 = call-poly <vilib>:"Create Timing Source.vi"() -> ("name (out)"=w132:string)  [unwired: 10 in, 1 out]
        n15 = while {
          tunnel: w135 -> [w393]
          tunnel: w134 -> [w392]
          tunnel: w133 -> [w391]
          tunnel: w132 -> [w384]
          tunnel: w131 -> [w377]
          tunnel: w130 -> [w376]
          tunnel: [w372] -> w129
          tunnel: [w371] -> w128
          tunnel: [w369] -> w127
          tunnel: [w367] -> w126
          tunnel: [w365] -> w125
          tunnel: [w363] -> w124
          shift-right: [w336] -> _
          shift-left: dbl[] [] -> [w341]
          shift-right: [w314] -> _
          shift-left: dbl[] [] -> [w349]
          shift-right: [w338] -> _
          shift-left: dbl[] [] -> [w345]
          shift-right: [w311] -> _
          shift-left: dbl[] [] -> [w348]
          shift-right: [w308] -> _
          shift-left: dbl[] [] -> [w347]
          tunnel: w118 -> [w302]
          tunnel: w117 -> [w258]
          tunnel: w116 -> [w254]
          shift-right: [w212] -> _
          shift-left: dbl[] [] -> [w242]
          shift-right: [w210] -> _
          shift-left: dbl[] [] -> [w240]
          shift-right: [w208] -> _
          shift-left: dbl[] [] -> [w238]
          shift-right: [w206] -> _
          shift-left: dbl[] [] -> [w236]
          tunnel: ["stop"] -> w111
          tunnel: [w200] -> w110
          tunnel: w109 -> [w195]
          tunnel: w108 -> [w193]
          tunnel: w107 -> [w173]
          tunnel: w106 -> [w172]
          shift-right: [w137] -> _
          shift-left: dbl[] [] -> [w163]
          shift-right: [w145] -> _
          shift-left: dbl[] [] -> [w157]
          shift-right: [w141] -> _
          shift-left: dbl[] [] -> [w152]
          stop <- w199 stop-if-true
          n16 = flat-sequence {
            tunnel: w302 -> [w407]
            tunnel: w341 -> [w408]
            tunnel: w345 -> [w409]
            tunnel: w347 -> [w410]
            tunnel: w348 -> [w411]
            tunnel: w349 -> [w412]
            tunnel: w376 -> [w413]
            tunnel: w377 -> [w414]
            tunnel: w391 -> [w415]
            tunnel: w392 -> [w416]
            tunnel: w393 -> [w417]
            tunnel: [w417] -> w301
            tunnel: [w416] -> w300
            tunnel: [w415] -> w299
            tunnel: [w414] -> w298
            tunnel: [w413] -> w297
            tunnel: [w412] -> w296
            tunnel: [w411] -> w295
            tunnel: [w410] -> w294
            tunnel: [w409] -> w293
            tunnel: [w408] -> w292
            tunnel: [w407] -> w291
            tunnel: [w406] -> w273
            tunnel: [w405] -> w259
            tunnel: w258 -> [w405]
            tunnel: [w404] -> w255
            tunnel: w254 -> [w404]
            tunnel: [w403] -> w243
            tunnel: w242 -> [w403]
            tunnel: [w402] -> w241
            tunnel: w240 -> [w402]
            tunnel: [w401] -> w239
            tunnel: w238 -> [w401]
            tunnel: [w400] -> w237
            tunnel: w236 -> [w400]
            tunnel: [w399] -> w196
            tunnel: w195 -> [w399]
            tunnel: [w398] -> w194
            tunnel: w193 -> [w398]
            tunnel: [w397] -> w174
            tunnel: w173 -> [w397]
            tunnel: [w396] -> w164
            tunnel: w163 -> [w396]
            tunnel: [w395] -> w158
            tunnel: w157 -> [w395]
            tunnel: [w394] -> w153
            tunnel: w152 -> [w394]
            tunnel: [w446] -> w390
            tunnel: [w445] -> w388
            tunnel: [w441] -> w386
            tunnel: [w440] -> w381
            tunnel: [w439] -> w379
            tunnel: [w438] -> w346
            tunnel: [w437] -> w342
            tunnel: [w436] -> w322
            tunnel: [w435] -> w319
            tunnel: [w434] -> w317
            tunnel: [w433] -> w303
            tunnel: w301 -> [w446]
            tunnel: w300 -> [w445]
            tunnel: w299 -> [w444]
            tunnel: w298 -> [w440]
            tunnel: w297 -> [w439]
            tunnel: w296 -> [w436]
            tunnel: w295 -> [w435]
            tunnel: w294 -> [w434]
            tunnel: w293 -> [w438]
            tunnel: w292 -> [w437]
            tunnel: w291 -> [w433]
            tunnel: [w432] -> w274
            tunnel: w273 -> [w432]
            tunnel: w259 -> [w430]
            tunnel: [w430] -> w256
            tunnel: w255 -> [w431]
            tunnel: [w431] -> w252
            tunnel: w243 -> [w429]
            tunnel: w241 -> [w428]
            tunnel: w239 -> [w427]
            tunnel: w237 -> [w426]
            tunnel: [w429] -> w235
            tunnel: [w428] -> w231
            tunnel: [w427] -> w228
            tunnel: [w426] -> w227
            tunnel: w196 -> [w425]
            tunnel: w194 -> [w424]
            tunnel: [w425] -> w191
            tunnel: [w424] -> w189
            tunnel: w174 -> [w423]
            tunnel: w172 -> [w422]
            tunnel: [w421] -> w165
            tunnel: w164 -> [w421]
            tunnel: [w420] -> w159
            tunnel: w158 -> [w420]
            tunnel: [w419] -> w154
            tunnel: w153 -> [w419]
            tunnel: [w418] -> w148
            tunnel: w390 -> [w1162]
            tunnel: [w1162] -> w389
            tunnel: w388 -> [w1161]
            tunnel: [w1161] -> w387
            tunnel: w386 -> [w1157]
            tunnel: [w1157] -> w385
            tunnel: w384 -> [w1158]
            tunnel: [w1158] -> w383
            tunnel: [w1158] -> w382
            tunnel: w381 -> [w1160]
            tunnel: [w1160] -> w380
            tunnel: w379 -> [w1159]
            tunnel: [w1159] -> w378
            tunnel: [w1158] -> w375
            tunnel: [w1158] -> w361
            tunnel: w346 -> [w1156]
            tunnel: [w1156] -> w344
            tunnel: w342 -> [w1155]
            tunnel: [w1155] -> w339
            tunnel: [w1154] -> w323
            tunnel: w322 -> [w1154]
            tunnel: [w1153] -> w320
            tunnel: w319 -> [w1153]
            tunnel: [w1152] -> w318
            tunnel: w317 -> [w1152]
            tunnel: [w1151] -> w304
            tunnel: w303 -> [w1151]
            tunnel: [w1150] -> w275
            tunnel: w274 -> [w1150]
            tunnel: [w1149] -> w257
            tunnel: w256 -> [w1149]
            tunnel: [w1148] -> w253
            tunnel: w252 -> [w1148]
            tunnel: w235 -> [w1147]
            tunnel: [w1147] -> w234
            tunnel: [w1146] -> w232
            tunnel: w231 -> [w1146]
            tunnel: [w1145] -> w230
            tunnel: w228 -> [w1145]
            tunnel: w227 -> [w1144]
            tunnel: [w1144] -> w226
            tunnel: [w1143] -> w192
            tunnel: w191 -> [w1143]
            tunnel: [w1142] -> w190
            tunnel: w189 -> [w1142]
            tunnel: [w1141] -> w166
            tunnel: w165 -> [w1141]
            tunnel: [w1140] -> w160
            tunnel: w159 -> [w1140]
            tunnel: [w1139] -> w155
            tunnel: w154 -> [w1139]
            tunnel: [w1138] -> w149
            tunnel: w148 -> [w1138]
            tunnel: [w1193] -> w360
            tunnel: w389 -> [w1222]
            tunnel: w387 -> [w1221]
            tunnel: w385 -> [w1218]
            tunnel: w383 -> [w1217]
            tunnel: w382 -> [w1216]
            tunnel: w380 -> [w1206]
            tunnel: w378 -> [w1205]
            tunnel: w375 -> [w1207]
            tunnel: [w1203] -> w359
            tunnel: [w1204] -> w358
            tunnel: [w1215] -> w357
            tunnel: [w1214] -> w356
            tunnel: [w1213] -> w355
            tunnel: [w1212] -> w354
            tunnel: w361 -> [w1202]
            tunnel: [w1201] -> w353
            tunnel: [w1200] -> w352
            tunnel: [w1184] -> w351
            tunnel: [w1199] -> w350
            tunnel: w344 -> [w1198]
            tunnel: [w1198] -> w343
            tunnel: [w1197] -> w340
            tunnel: w339 -> [w1197]
            tunnel: w323 -> [w1196]
            tunnel: [w1196] -> w321
            tunnel: w320 -> [w1195]
            tunnel: w318 -> [w1194]
            tunnel: [w1195] -> w316
            tunnel: [w1194] -> w315
            tunnel: w304 -> [w1192]
            tunnel: [w1188] -> w276
            tunnel: w275 -> [w1188]
            tunnel: w257 -> [w1186]
            tunnel: w253 -> [w1185]
            tunnel: [w1179] -> w251
            tunnel: [w1184] -> w250
            tunnel: [w1182] -> w249
            tunnel: [w1180] -> w248
            tunnel: w234 -> [w1183]
            tunnel: [w1183] -> w233
            tunnel: w232 -> [w1182]
            tunnel: w230 -> [w1181]
            tunnel: [w1181] -> w229
            tunnel: w226 -> [w1180]
            tunnel: [w1179] -> w204
            tunnel: [w1178] -> w201
            tunnel: w192 -> [w1177]
            tunnel: w190 -> [w1176]
            tunnel: [w1173] -> w185
            tunnel: [w1171] -> w184
            tunnel: [w1173] -> w183
            tunnel: [w1172] -> w179
            tunnel: [w1171] -> w176
            tunnel: [w1170] -> w167
            tunnel: w166 -> [w1170]
            tunnel: [w1169] -> w162
            tunnel: [w1168] -> w161
            tunnel: w160 -> [w1168]
            tunnel: [w1167] -> w156
            tunnel: w155 -> [w1167]
            tunnel: [w1166] -> w151
            tunnel: [w1165] -> w150
            tunnel: w149 -> [w1164]
            tunnel: w360 -> [w1474]
            tunnel: [w1471] -> w334
            tunnel: w359 -> [w1487]
            tunnel: [w1487] -> w333
            tunnel: w358 -> [w1486]
            tunnel: [w1486] -> w332
            tunnel: w357 -> [w1485]
            tunnel: [w1485] -> w331
            tunnel: w356 -> [w1484]
            tunnel: [w1484] -> w330
            tunnel: w355 -> [w1483]
            tunnel: [w1483] -> w329
            tunnel: w354 -> [w1482]
            tunnel: [w1482] -> w328
            tunnel: [w1475] -> w327
            tunnel: w353 -> [w1468]
            tunnel: w352 -> [w1476]
            tunnel: w351 -> [w1475]
            tunnel: w350 -> [w1477]
            tunnel: [w1474] -> w326
            tunnel: w343 -> [w1473]
            tunnel: w340 -> [w1472]
            tunnel: [w1470] -> w325
            tunnel: [w1458] -> w324
            tunnel: w321 -> [w1469]
            tunnel: w316 -> [w1466]
            tunnel: w315 -> [w1465]
            tunnel: [w1467] -> w312
            tunnel: [w1464] -> w309
            tunnel: [w1463] -> w306
            tunnel: [w1459] -> w305
            tunnel: [w1457] -> w277
            tunnel: w276 -> [w1457]
            tunnel: w251 -> [w1456]
            tunnel: w250 -> [w1455]
            tunnel: w249 -> [w1454]
            tunnel: w248 -> [w1452]
            tunnel: [w1450] -> w247
            tunnel: [w1449] -> w246
            tunnel: [w1448] -> w245
            tunnel: [w1447] -> w244
            tunnel: w233 -> [w1451]
            tunnel: w229 -> [w1453]
            tunnel: [w1450] -> w225
            tunnel: [w1449] -> w224
            tunnel: [w1448] -> w223
            tunnel: [w1447] -> w222
            tunnel: [w1446] -> w205
            tunnel: w204 -> [w1446]
            tunnel: [w1445] -> w202
            tunnel: w201 -> [w1445]
            tunnel: w185 -> [w1444]
            tunnel: w184 -> [w1443]
            tunnel: w183 -> [w1442]
            tunnel: [w1442] -> w182
            tunnel: [w1441] -> w180
            tunnel: w179 -> [w1441]
            tunnel: w176 -> [w1440]
            tunnel: [w1440] -> w175
            tunnel: [w1438] -> w168
            tunnel: w167 -> [w1439]
            tunnel: w162 -> [w1431]
            tunnel: w161 -> [w1437]
            tunnel: w156 -> [w1436]
            tunnel: w151 -> [w1432]
            tunnel: w150 -> [w1433]
            tunnel: [w1435] -> w147
            tunnel: [w1434] -> w146
            tunnel: [w1430] -> w136
            tunnel: w334 -> [w1520]
            tunnel: [w1527] -> w374
            tunnel: [w1526] -> w373
            tunnel: w333 -> [w1526]
            tunnel: [w1521] -> w370
            tunnel: w332 -> [w1521]
            tunnel: [w1525] -> w368
            tunnel: w331 -> [w1525]
            tunnel: [w1524] -> w366
            tunnel: w330 -> [w1524]
            tunnel: [w1523] -> w364
            tunnel: w329 -> [w1523]
            tunnel: [w1522] -> w362
            tunnel: w328 -> [w1522]
            tunnel: w327 -> [w1494]
            tunnel: w326 -> [w1515]
            tunnel: w325 -> [w1499]
            tunnel: [w1499] -> w337
            tunnel: w324 -> [w1491]
            tunnel: [w1491] -> w335
            tunnel: [w1517] -> w313
            tunnel: w312 -> [w1517]
            tunnel: [w1518] -> w310
            tunnel: w309 -> [w1518]
            tunnel: [w1519] -> w307
            tunnel: w306 -> [w1519]
            tunnel: w305 -> [_]
            tunnel: [w1514] -> w278
            tunnel: w277 -> [w1514]
            tunnel: w247 -> [w1513]
            tunnel: w246 -> [w1512]
            tunnel: w245 -> [w1511]
            tunnel: w244 -> [w1510]
            tunnel: w225 -> [w1509]
            tunnel: w224 -> [w1508]
            tunnel: w223 -> [w1507]
            tunnel: w222 -> [w1506]
            tunnel: [w1509] -> w220
            tunnel: [w1508] -> w218
            tunnel: [w1507] -> w216
            tunnel: [w1506] -> w214
            tunnel: w205 -> [_]
            tunnel: [w1505] -> w203
            tunnel: w202 -> [w1505]
            tunnel: w182 -> [_]
            tunnel: [w1503] -> w181
            tunnel: w180 -> [w1503]
            tunnel: w175 -> [_]
            tunnel: [w1492] -> w169
            tunnel: w168 -> [w1492]
            tunnel: w147 -> [w1497]
            tunnel: w146 -> [w1498]
            tunnel: [w1498] -> w142
            tunnel: [w1497] -> w138
            tunnel: w136 -> [w1495]
            tunnel: w374 -> [w1543]
            tunnel: w373 -> [w1558]
            tunnel: w370 -> [w1552]
            tunnel: w368 -> [w1557]
            tunnel: w366 -> [w1554]
            tunnel: w364 -> [w1556]
            tunnel: w362 -> [w1555]
            tunnel: w337 -> [w1548]
            tunnel: w335 -> [w1547]
            tunnel: w313 -> [w1546]
            tunnel: w310 -> [w1545]
            tunnel: w307 -> [w1544]
            tunnel: [w1537] -> w198
            tunnel: [w1558] -> w290
            tunnel: [w1552] -> w289
            tunnel: [w1557] -> w288
            tunnel: [w1554] -> w287
            tunnel: [w1556] -> w286
            tunnel: [w1555] -> w285
            tunnel: [w1548] -> w284
            tunnel: [w1547] -> w283
            tunnel: [w1546] -> w282
            tunnel: [w1545] -> w281
            tunnel: [w1544] -> w280
            tunnel: [w1542] -> w279
            tunnel: w278 -> [w1542]
            tunnel: [w1541] -> w221
            tunnel: w220 -> [w1541]
            tunnel: [w1540] -> w219
            tunnel: w218 -> [w1540]
            tunnel: [w1539] -> w217
            tunnel: w216 -> [w1539]
            tunnel: [w1538] -> w215
            tunnel: w214 -> [w1538]
            tunnel: w203 -> [w1536]
            tunnel: [w1535] -> w188
            tunnel: [w1534] -> w187
            tunnel: w181 -> [w1533]
            tunnel: [w1532] -> w178
            tunnel: [w1531] -> w177
            tunnel: [w1530] -> w170
            tunnel: w169 -> [w1530]
            tunnel: [w1529] -> w143
            tunnel: w142 -> [w1529]
            tunnel: [w1528] -> w139
            tunnel: w138 -> [w1528]
            tunnel: w290 -> [w1608]
            tunnel: w289 -> [w1607]
            tunnel: w288 -> [w1606]
            tunnel: w287 -> [w1605]
            tunnel: w286 -> [w1604]
            tunnel: w285 -> [w1603]
            tunnel: w284 -> [w1602]
            tunnel: w283 -> [w1601]
            tunnel: w282 -> [w1600]
            tunnel: w281 -> [w1599]
            tunnel: w280 -> [w1598]
            tunnel: w279 -> [w1591]
            tunnel: [w1608] -> w272
            tunnel: [w1607] -> w271
            tunnel: [w1606] -> w270
            tunnel: [w1605] -> w269
            tunnel: [w1604] -> w268
            tunnel: [w1603] -> w267
            tunnel: [w1602] -> w266
            tunnel: [w1601] -> w265
            tunnel: [w1600] -> w264
            tunnel: [w1599] -> w263
            tunnel: [w1598] -> w262
            tunnel: [w1591] -> w261
            tunnel: [w1590] -> w260
            tunnel: w221 -> [w1588]
            tunnel: w219 -> [w1587]
            tunnel: w217 -> [w1586]
            tunnel: w215 -> [w1585]
            tunnel: [w1588] -> w213
            tunnel: [w1587] -> w211
            tunnel: [w1586] -> w209
            tunnel: [w1585] -> w207
            tunnel: w188 -> [w1584]
            tunnel: w187 -> [w1583]
            tunnel: [w1578] -> w186
            tunnel: w178 -> [w1577]
            tunnel: w177 -> [w1576]
            tunnel: [w1575] -> w171
            tunnel: w170 -> [w1575]
            tunnel: [w1574] -> w144
            tunnel: w143 -> [w1574]
            tunnel: [w1573] -> w140
            tunnel: w139 -> [w1573]
            tunnel: [w1622] -> w308
            tunnel: [w1623] -> w311
            tunnel: [w1624] -> w314
            tunnel: [w1625] -> w336
            tunnel: [w1626] -> w338
            tunnel: [w1627] -> w363
            tunnel: [w1628] -> w365
            tunnel: [w1629] -> w367
            tunnel: [w1630] -> w369
            tunnel: [w1631] -> w371
            tunnel: [w1632] -> w372
            tunnel: w272 -> [w1632]
            tunnel: w271 -> [w1631]
            tunnel: w270 -> [w1630]
            tunnel: w269 -> [w1629]
            tunnel: w268 -> [w1628]
            tunnel: w267 -> [w1627]
            tunnel: w266 -> [w1626]
            tunnel: w265 -> [w1625]
            tunnel: w264 -> [w1624]
            tunnel: w263 -> [w1623]
            tunnel: w262 -> [w1622]
            tunnel: w261 -> [w1618]
            tunnel: w260 -> [w1617]
            tunnel: [w1616] -> w212
            tunnel: w213 -> [w1616]
            tunnel: [w1615] -> w210
            tunnel: w211 -> [w1615]
            tunnel: [w1614] -> w208
            tunnel: w209 -> [w1614]
            tunnel: [w1613] -> w206
            tunnel: w207 -> [w1613]
            tunnel: [w1612] -> w200
            tunnel: w186 -> [w1612]
            tunnel: [w1611] -> w137
            tunnel: w171 -> [w1611]
            tunnel: [w1610] -> w145
            tunnel: w144 -> [w1610]
            tunnel: [w1609] -> w141
            tunnel: w140 -> [w1609]
            frame #0 {
              n17 = Tick Count (ms)() -> (millisecond timer value=w406:u32)
            }
            frame #1 {
              n18 = while {
                tunnel: w444 -> [w454]
                tunnel: [w453] -> w443
                tunnel: [w452] -> w442
                tunnel: w430 -> [w450]
                tunnel: w423 -> [w449]
                tunnel: w422 -> [w448]
                tunnel: [w447] -> w418
                stop <- w455 stop-if-true
                n19 = event shown="[4] \"Reset STOPP\": Value Change" {
                  selector: _ -> [_ _ _ _ _ _ _ _ _ _ _ _ _ _ _]
                  dyn-events: _ -> [_ _ _ _ _ _ _ _ _ _ _ _ _ _ _]
                  timeout: 1 -> [_ _ _ _ _ _ _ _ _ _ _ _ _ _ _]
                  tunnel: [TRUE ("Set Gauge to Zero") w465 w515 w537 w564 "Set Value" w677 w734 w786 w866 w938 "Set Gauge to Zero" w1029 "Get SetPoint" _] -> w455
                  tunnel: w454 -> [w460 w464 w512 w535 w560 w638 w676 w730 w784 w864 w936 w1014 w1032 w1118 w1132]
                  tunnel: [w459 w463 w511 w534 w562 w637 w674 w732 w783 w863 w935 w1013 w1031 w1116 w1131] -> w453
                  tunnel: [w458 w462 w510 w533 w561 w634 w675 w731 w782 w862 w934 w1012 w1030 w1114 w1130] -> w452
                  tunnel: w450 -> [_ _ _ _ _ _ _ _ _ _ _ w1010 _ _ _]
                  tunnel: w449 -> [w456 w461 w509 w532 w559 w636 w673 w729 w781 w861 w933 w1005 w1033 w1115 w1124]
                  tunnel: w448 -> [_ _ _ _ _ w635 _ _ _ _ _ _ _ _ _]
                  tunnel: [w456 w461 w509 w532 w559 w633 w673 w729 w781 w861 w933 w1005 w1033 w1115 w1124] -> w447
                  event Timeout {
                    n20 = event-data() -> ()  [unwired: 1 in, 1 out]
                    n21 = Unbundle(w460) -> ("VISA resource name out"=w459:refnum<visa-resource-name>, "error out"=w458:errorcluster)  [unwired: 2 out]
                  }
                  event "START": Value Change {
                    n22 = event-data() -> ()  [unwired: 1 in, 1 out]
                    n23 = stacked-sequence {
                      tunnel: w464 -> [_ w471 _]
                      tunnel: [_ w470 _] -> w462
                      tunnel: [_ w469 _] -> w463
                      frame #0 {
                        n24 = property on="START" class="Bool"("Blinking"=TRUE) -> ()  [unwired: 2 in, 2 out]
                        n25 = property on="ON" class="Bool (strict)"("Blinking"=FALSE) -> ()  [unwired: 2 in, 2 out]
                      }
                      frame #1 {
                        n26 = for {
                          N: 2 -> [_]
                          tunnel: w471 -> [w475]
                          tunnel: [w474] -> w470
                          tunnel: [w473] -> w469
                          i -> [w477]
                          n27 = flat-sequence {
                            tunnel: [w480] -> w476
                            tunnel: w477 -> [w479]
                            tunnel: [w498] -> w478
                            tunnel: w476 -> [w497]
                            tunnel: w475 -> [w499]
                            tunnel: [w496] -> w474
                            tunnel: [w495] -> w473
                            tunnel: w478 -> [w505]
                            tunnel: w477 -> [w504]
                            frame #0 {
                              n28 = case shown="0, Default" w479 {
                                tunnel: [w489 w491] -> w480
                                frame 0, Default {
                                n29 = Multiply(x=10.0, y="SP 1 input (°C)") -> (x*y=w486:dbl)
                                n30 = local read "RAM"() -> (w484:bool)
                                n31 = Number To Hexadecimal String(1:i16 5 ("width (-)"), 2:w486) -> (0:w488:string)
                                n32 = Select(t="*P012", s=w484, f="*P012") -> (s? t:f=w481:string)
                                n33 = Concatenate Strings(w481, w488) -> (w489:string)
                                }
                                frame 1 {
                                n34 = local read "RAM"() -> (w494:bool)
                                n35 = Select(t="*G01", s=w494, f="*R01") -> (s? t:f=w491:string)
                                }
                              }
                            }
                            frame #1 {
                              n36 = Unbundle(w499) -> ("VISA resource name out"=w500:refnum<visa-resource-name>, "error out"=w502:errorcluster, "Delay (ms)"=w501:u32, "Write/\nRead"=w503:bool)
                              n37 = call "I3252_Comm_Interface.vi"("VISA resource name in"=w500, "error in"=w502, "Delay (ms)"=w501, "Write"=w503, "String to Write"=w497, "Read"=w503) -> ("VISA resource name out"=w495:refnum<visa-resource-name>, "error out"=w496:errorcluster, "Read String"=w498:string)  [unwired: 2 in]
                            }
                            frame #2 {
                              n38 = case shown="1" w504 {
                                tunnel: w505 -> [_ w507]
                                frame 0, Default {
                                }
                                frame 1 {
                                n39 = call "I3252_Edit_Setpoint.vi"("Read String"=w507) -> ("Setpoint is"=→"SP 1 is (°C)":dbl)
                                }
                              }
                            }
                          }
                        }
                      }
                      frame #2 {
                        n40 = property on="START" class="Bool"("Blinking"=FALSE) -> ()  [unwired: 2 in, 2 out]
                      }
                    }
                    n41 = Not(x="START") -> (.not. x?=w465:bool)
                  }
                  event "Standby": Value Change {
                    n42 = event-data() -> ()  [unwired: 1 in, 1 out]
                    n43 = flat-sequence {
                      tunnel: [w523] -> w513
                      tunnel: w513 -> [w527]
                      tunnel: w512 -> [w526]
                      tunnel: [w525] -> w510
                      tunnel: [w524] -> w511
                      frame #0 {
                        n44 = local read "Standby"() -> (w516:bool)
                        n45 = Select(t=TRUE, s=w516, f=FALSE) -> (s? t:f=w519:bool)
                        n46 = property on="Standby" class="Bool (strict)"("Blinking"=w519) -> ()  [unwired: 2 in, 2 out]
                      }
                      frame #1 {
                        n47 = local read "Standby"() -> (w521:bool)
                        n48 = Select(t="*D03", s=w521, f="*E03") -> (s? t:f=w523:string)
                      }
                      frame #2 {
                        n49 = Unbundle(w526) -> ("VISA resource name out"=w528:refnum<visa-resource-name>, "error out"=w530:errorcluster, "Delay (ms)"=w529:u32, "Write/\nRead"=w531:bool)
                        n50 = call "I3252_Comm_Interface.vi"("VISA resource name in"=w528, "error in"=w530, "Delay (ms)"=w529, "Write"=w531, "String to Write"=w527, "Read"=w531) -> ("VISA resource name out"=w524:refnum<visa-resource-name>, "error out"=w525:errorcluster)  [unwired: 2 in, 1 out]
                      }
                    }
                    n51 = Not(x="Standby") -> (.not. x?=w515:bool)
                  }
                  event "Set Command": Value Change {
                    n52 = event-data() -> ()  [unwired: 1 in, 1 out]
                    n53 = stacked-sequence {
                      tunnel: w535 -> [_ w542 _]
                      tunnel: [_ w541 _] -> w534
                      tunnel: [_ w540 _] -> w533
                      frame #0 {
                        n54 = property on="Set Command" class="Bool"("Blinking"=TRUE) -> ()  [unwired: 2 in, 2 out]
                        n55 = property on="ON" class="Bool (strict)"("Blinking"=FALSE) -> ()  [unwired: 2 in, 2 out]
                      }
                      frame #1 {
                        n56 = flat-sequence {
                          tunnel: [w547] -> w544
                          tunnel: [w550] -> w543
                          tunnel: w544 -> [w551]
                          tunnel: w542 -> [w552]
                          tunnel: [w549] -> w541
                          tunnel: [w548] -> w540
                          tunnel: w543 -> [w557]
                          frame #0 {
                            n57 = Concatenate Strings("*", "Command input") -> (w547:string)
                          }
                          frame #1 {
                            n58 = Unbundle(w552) -> ("VISA resource name out"=w556:refnum<visa-resource-name>, "error out"=w554:errorcluster, "Delay (ms)"=w555:u32, "Write/\nRead"=w553:bool)
                            n59 = call "I3252_Comm_Interface.vi"("VISA resource name in"=w556, "error in"=w554, "Delay (ms)"=w555, "Write"=w553, "String to Write"=w551, "Read"=w553) -> ("VISA resource name out"=w549:refnum<visa-resource-name>, "error out"=w548:errorcluster, "Read String"=w550:string)  [unwired: 2 in]
                          }
                          frame #2 {
                            "Command output" <- w557
                          }
                        }
                      }
                      frame #2 {
                        n60 = property on="Set Command" class="Bool"("Blinking"=FALSE) -> ()  [unwired: 2 in, 2 out]
                      }
                    }
                    n61 = Not(x="Set Command") -> (.not. x?=w537:bool)
                  }
                  event "Reset\nSTOPP": Value Change {
                    n62 = event-data() -> ()  [unwired: 1 in, 1 out]
                    n63 = stacked-sequence {
                      tunnel: [_ _ w606 _] -> w561
                      tunnel: [_ _ w605 _] -> w562
                      tunnel: w560 -> [_ w568 w603 _]
                      frame #0 {
                        n64 = property on="Reset\nSTOPP" class="Bool"("Blinking"=FALSE) -> ()  [unwired: 2 in, 2 out]
                        n65 = property on="ON" class="Bool (strict)"("Blinking"=FALSE) -> ()  [unwired: 2 in, 2 out]
                      }
                      frame #1 {
                        n66 = property on="RAMP" class="Bool (strict)"() -> ("Value"=w567:bool)  [unwired: 2 in, 2 out]
                        n67 = case shown="True" w567 {
                          tunnel: w568 -> [_ w571]
                          frame False {
                          }
                          frame True {
                            n68 = property on="RAMP" class="Bool (strict)"("Value"=FALSE ("RAMP")) -> ()  [unwired: 2 in, 2 out]
                            n69 = for {
                              N: 5 -> [_]
                              tunnel: [w577] -> _
                              tunnel: [w576] -> _
                              tunnel: w571 -> [w575]
                              i -> [w573]
                              n70 = flat-sequence {
                                tunnel: w573 -> [w579]
                                tunnel: [w578] -> w574
                                tunnel: [w595] -> w577
                                tunnel: [w596] -> w576
                                tunnel: w575 -> [w597]
                                tunnel: w574 -> [w594]
                                frame #0 {
                                n71 = case shown="0, Default" w579 {
                                tunnel: ["*D03" w583 w586 w590 "*E03" ("string") "*Z02" ("string")] -> w578
                                frame 0, Default {
                                }
                                frame 1 {
                                n72 = Select(t="*W0D78", s=FALSE, f="*W0D60") -> (s? t:f=w583:string)
                                }
                                frame 2 {
                                n73 = case shown="True" FALSE {
                                tunnel: ["*W0E0000" ("string") ""] -> w586
                                frame False {
                                }
                                frame True {
                                }
                                }
                                }
                                frame 3 {
                                n74 = case shown="False" FALSE {
                                tunnel: ["*W1E0000" ("string") _] -> w590
                                frame False {
                                }
                                frame True {
                                }
                                }
                                }
                                frame 4 {
                                }
                                frame 5 {
                                }
                                }
                                }
                                frame #1 {
                                n75 = Unbundle(w597) -> ("VISA resource name out"=w598:refnum<visa-resource-name>, "error out"=w600:errorcluster, "Delay (ms)"=w599:u32, "Write/\nRead"=w601:bool)
                                n76 = call "I3252_Comm_Interface.vi"("VISA resource name in"=w598, "error in"=w600, "Delay (ms)"=w599, "Write"=w601, "String to Write"=w594, "Read"=w601) -> ("VISA resource name out"=w596:refnum<visa-resource-name>, "error out"=w595:errorcluster)  [unwired: 2 in, 1 out]
                                }
                              }
                              n77 = Wait (ms)(milliseconds to wait=u32 1000) -> ()  [unwired: 1 out]
                            }
                          }
                        }
                      }
                      frame #2 {
                        n78 = for {
                          N: 2 -> [_]
                          tunnel: [w612] -> w606
                          tunnel: [w611] -> w605
                          tunnel: w603 -> [w610]
                          i -> [w608]
                          n79 = flat-sequence {
                            tunnel: w608 -> [w614]
                            tunnel: [w613] -> w609
                            tunnel: [w619] -> w612
                            tunnel: [w620] -> w611
                            tunnel: w610 -> [w621]
                            tunnel: w609 -> [w618]
                            tunnel: [w617] -> w607
                            tunnel: w608 -> [w627]
                            tunnel: w607 -> [w626]
                            frame #0 {
                              n80 = case shown="1" w614 {
                                tunnel: ["*Z02" "*G01"] -> w613
                                frame 0, Default {
                                }
                                frame 1 {
                                }
                              }
                            }
                            frame #1 {
                              n81 = Unbundle(w621) -> ("VISA resource name out"=w622:refnum<visa-resource-name>, "error out"=w624:errorcluster, "Delay (ms)"=w623:u32, "Write/\nRead"=w625:bool)
                              n82 = call "I3252_Comm_Interface.vi"("VISA resource name in"=w622, "error in"=w624, "Delay (ms)"=w623, "Write"=w625, "String to Write"=w618, "Read"=w625) -> ("VISA resource name out"=w620:refnum<visa-resource-name>, "error out"=w619:errorcluster, "Read String"=w617:string)  [unwired: 2 in]
                            }
                            frame #2 {
                              n83 = case shown="1" w627 {
                                tunnel: w626 -> [_ w629]
                                frame 0, Default {
                                }
                                frame 1 {
                                n84 = call "I3252_Edit_Setpoint.vi"("Read String"=w629) -> ("Setpoint is"=w628:dbl)
                                n85 = local write "SP 1 is (°C)"(w628) -> ()
                                }
                              }
                            }
                          }
                        }
                        n86 = Wait (ms)(milliseconds to wait=u32 4000) -> ()  [unwired: 1 out]
                      }
                      frame #3 {
                        n87 = property on="Reset\nSTOPP" class="Bool"("Blinking"=FALSE) -> ()  [unwired: 2 in, 2 out]
                      }
                    }
                    n88 = Not(x="Reset\nSTOPP") -> (.not. x?=w564:bool)
                  }
                  event "Set Value": Value Change {
                    n89 = event-data() -> ()  [unwired: 1 in, 4 out]
                    n90 = case shown="True" "OUTPUT" {
                      tunnel: w636 -> [w642 w647]
                      tunnel: w635 -> [w640 w646]
                      tunnel: [w639 w645] -> w634
                      tunnel: [w641 w644] -> w633
                      frame False {
                        n91 = VISA Write(VISA resource name=w642, write buffer=" :OUTP OFF;" ("string"), error in (no error)=w640) -> (VISA resource name out=w641:refnum<visa-resource-name>, error out=w639:errorcluster)  [unwired: 1 out]
                      }
                      frame True {
                        n92 = case shown="\"2\", Default" "Unit" {
                          tunnel: [1e-09 ("y") 1e-06 ("y") 0.001 ("y")] -> w655
                          frame "2", Default {
                          }
                          frame "1" {
                          }
                          frame "0" {
                          }
                        }
                        n93 = case shown="\"1\", Default" "Unit   2" {
                          tunnel: [0.001 ("y") 1.0 ("y")] -> w651
                          frame "1", Default {
                          }
                          frame "0" {
                          }
                        }
                        n94 = Multiply(x="Source \nCurrent", y=w655) -> (x*y=w658:dbl)
                        n95 = Multiply(x="Voltage\nCompl.", y=w651) -> (x*y=w649:dbl)
                        n96 = Number To Exponential String(number=w658, 1:FALSE ("use system decimal point (T)")) -> (E-format string=w660:string)  [unwired: 2 in]
                        n97 = Concatenate Strings(":SOUR:CURR " ("string"), w660) -> (w666:string)
                        n98 = Number To Exponential String(number=w649, 1:FALSE ("use system decimal point (T)")) -> (E-format string=w653:string)  [unwired: 2 in]
                        n99 = Concatenate Strings(" ;:VOLT:PROT " ("string"), w653) -> (w665:string)
                        n100 = Concatenate Strings(":SYST:RSEN ON;:SOUR:CURR:RANG:AUTO 1 ;:SOUR:FUNC CURR ;" ("write buffer"), w666, w665, " ;:OUTP ON" ("string"), "\r") -> (w664:string)
                        n101 = VISA Write(VISA resource name=w647, write buffer=w664, error in (no error)=w646) -> (VISA resource name out=w644:refnum<visa-resource-name>, error out=w645:errorcluster)  [unwired: 1 out]
                      }
                    }
                    n102 = Unbundle(w638) -> ("VISA resource name out"=w637:refnum<visa-resource-name>)  [unwired: 3 out]
                  }
                  event "Auto Tune": Value Change {
                    n103 = event-data() -> ()  [unwired: 1 in, 1 out]
                    n104 = stacked-sequence {
                      tunnel: w676 -> [_ w683 w728]
                      tunnel: [_ w682 _] -> w675
                      tunnel: [_ w681 _] -> w674
                      frame #0 {
                        n105 = property on="Auto Tune" class="Bool"("Blinking"=TRUE) -> ()  [unwired: 2 in, 2 out]
                        n106 = property on="ON" class="Bool (strict)"("Blinking"=FALSE) -> ()  [unwired: 2 in, 2 out]
                      }
                      frame #1 {
                        n107 = for {
                          N: 4 -> [_]
                          tunnel: [w688] -> w681
                          tunnel: [w687] -> w682
                          tunnel: w683 -> [w686]
                          i -> [w691]
                          n108 = flat-sequence {
                            tunnel: w691 -> [w693]
                            tunnel: [w692] -> w689
                            tunnel: w689 -> [w708]
                            tunnel: [w707] -> w690
                            tunnel: [w710] -> w688
                            tunnel: [w709] -> w687
                            tunnel: w686 -> [w706]
                            tunnel: w691 -> [w716]
                            tunnel: w690 -> [w715]
                            frame #0 {
                              n109 = case shown="2" w693 {
                                tunnel: ["*V01" w696 "*W0C35" "*Z02"] -> w692
                                frame 0, Default {
                                }
                                frame 1 {
                                n110 = local read "(°C)"() -> (w695:dbl)
                                n111 = Add(x=20.0, y=w695) -> (x+y=w702:dbl)
                                n112 = Multiply(x=10.0, y=w702) -> (x*y=w699:dbl)
                                n113 = Number To Hexadecimal String(1:i16 5 ("width (-)"), 2:w699) -> (0:w698:string)
                                n114 = Concatenate Strings("*W012", w698) -> (w696:string)
                                }
                                frame 2 {
                                # "35 hex = \n00110101 bin"
                                }
                                frame 3 {
                                }
                              }
                            }
                            frame #1 {
                              n115 = Unbundle(w706) -> ("VISA resource name out"=w714:refnum<visa-resource-name>, "error out"=w712:errorcluster, "Delay (ms)"=w713:u32, "Write/\nRead"=w711:bool)
                              n116 = call "I3252_Comm_Interface.vi"("VISA resource name in"=w714, "error in"=w712, "Delay (ms)"=w713, "Write"=w711, "String to Write"=w708, "Read"=w711) -> ("VISA resource name out"=w710:refnum<visa-resource-name>, "error out"=w709:errorcluster, "Read String"=w707:string)  [unwired: 2 in]
                            }
                            frame #2 {
                              n117 = case shown="0, Default" w716 {
                                tunnel: w715 -> [w718]
                                frame 0, Default {
                                n118 = call <vilib>:"Space Constant.vi"() -> ("String"=w721:string)
                                n119 = Search/Split String(string=w718, search string/char (-)=w721) -> (match + rest of string=w720:string)  [unwired: 1 in, 2 out]
                                n120 = Fract/Exp String To Number(use system decimal point (T)=FALSE, string=w720) -> (number=w717:dbl)  [unwired: 2 in, 1 out]
                                n121 = local write "(°C)"(w717) -> ()
                                }
                              }
                            }
                          }
                        }
                        n122 = Wait (ms)(milliseconds to wait=u32 45000) -> ()  [unwired: 1 out]
                      }
                      frame #2 {
                        n123 = Unbundle(w728) -> ("VISA resource name out"=w727:refnum<visa-resource-name>, "error out"=w725:errorcluster, "Delay (ms)"=w726:u32, "Write/\nRead"=w724:bool)
                        n124 = property on="Auto Tune" class="Bool"("Blinking"=FALSE) -> ()  [unwired: 2 in, 2 out]
                        n125 = call "I3252_Comm_Interface.vi"("VISA resource name in"=w727, "error in"=w725, "Delay (ms)"=w726, "Write"=w724, "String to Write"="*W01200000", "Read"=w724) -> ()  [unwired: 2 in, 3 out]
                      }
                    }
                    n126 = Not(x="Auto Tune") -> (.not. x?=w677:bool)
                  }
                  event "Write LOW/HI": Value Change {
                    n127 = event-data() -> ()  [unwired: 1 in, 1 out]
                    n128 = stacked-sequence {
                      tunnel: [_ w739 _] -> w732
                      tunnel: [_ w738 _] -> w731
                      tunnel: w730 -> [_ w737 _]
                      frame #0 {
                        n129 = property on="Write LOW/HI" class="Bool"("Blinking"=TRUE) -> ()  [unwired: 2 in, 2 out]
                        n130 = property on="ON" class="Bool (strict)"("Blinking"=FALSE) -> ()  [unwired: 2 in, 2 out]
                      }
                      frame #1 {
                        n131 = for {
                          N: 4 -> [_]
                          tunnel: [w743] -> w739
                          tunnel: [w742] -> w738
                          tunnel: w737 -> [w741]
                          i -> [w745]
                          n132 = flat-sequence {
                            tunnel: w745 -> [w747]
                            tunnel: [w748] -> w744
                            tunnel: w744 -> [w762]
                            tunnel: [w763] -> w746
                            tunnel: [w765] -> w743
                            tunnel: [w764] -> w742
                            tunnel: w741 -> [w761]
                            tunnel: w746 -> [w771]
                            tunnel: w745 -> [w770]
                            frame #0 {
                              n133 = case shown="0, Default" w747 {
                                tunnel: [w750 w756 "*R27" "*R28"] -> w748
                                frame 0, Default {
                                n134 = Number To Hexadecimal String(1:i16 2 ("width (-)"), 2:"% LOW Sollwert") -> (0:w751:string)
                                n135 = Concatenate Strings("*W27", w751) -> (w750:string)
                                }
                                frame 1 {
                                n136 = Number To Hexadecimal String(1:i16 2 ("width (-)"), 2:"% High Sollwert") -> (0:w757:string)
                                n137 = Concatenate Strings("*W28", w757) -> (w756:string)
                                }
                                frame 2 {
                                }
                                frame 3 {
                                }
                              }
                            }
                            frame #1 {
                              n138 = Unbundle(w761) -> ("VISA resource name out"=w769:refnum<visa-resource-name>, "error out"=w767:errorcluster, "Delay (ms)"=w768:u32, "Write/\nRead"=w766:bool)
                              n139 = call "I3252_Comm_Interface.vi"("VISA resource name in"=w769, "error in"=w767, "Delay (ms)"=w768, "Write"=w766, "String to Write"=w762, "Read"=w766) -> ("VISA resource name out"=w765:refnum<visa-resource-name>, "error out"=w764:errorcluster, "Read String"=w763:string)  [unwired: 2 in]
                            }
                            frame #2 {
                              n140 = case shown="0, Default" w770 {
                                tunnel: w771 -> [_ w775 w779]
                                frame 0, Default {
                                }
                                frame 2 {
                                n141 = String Subset(string=w775, offset (0)=3) -> (substring=w773:string)  [unwired: 1 in]
                                n142 = Hexadecimal String To Number(string=w773) -> (number=→"% LOW Istwert":u32)  [unwired: 2 in, 1 out]
                                }
                                frame 3 {
                                n143 = String Subset(string=w779, offset (0)=3) -> (substring=w777:string)  [unwired: 1 in]
                                n144 = Hexadecimal String To Number(string=w777) -> (number=→"% HIGH Istwert":u32)  [unwired: 2 in, 1 out]
                                }
                              }
                            }
                          }
                        }
                      }
                      frame #2 {
                        n145 = property on="Write LOW/HI" class="Bool"("Blinking"=FALSE) -> ()  [unwired: 2 in, 2 out]
                      }
                    }
                    n146 = Not(x="Write LOW/HI") -> (.not. x?=w734:bool)
                  }
                  event "Set PID": Value Change {
                    n147 = event-data() -> ()  [unwired: 1 in, 1 out]
                    n148 = stacked-sequence {
                      tunnel: w784 -> [_ w791 _]
                      tunnel: [_ w790 _] -> w783
                      tunnel: [_ w789 _] -> w782
                      frame #0 {
                        n149 = property on="Set PID" class="Bool"("Blinking"=TRUE) -> ()  [unwired: 2 in, 2 out]
                        n150 = property on="ON" class="Bool (strict)"("Blinking"=FALSE) -> ()  [unwired: 2 in, 2 out]
                      }
                      frame #1 {
                        n151 = for {
                          N: 6 -> [_]
                          tunnel: w791 -> [w795]
                          tunnel: [w794] -> w790
                          tunnel: [w793] -> w789
                          i -> [w797]
                          n152 = flat-sequence {
                            tunnel: w797 -> [w799]
                            tunnel: [w800] -> w796
                            tunnel: w796 -> [w841]
                            tunnel: [w837] -> w798
                            tunnel: w795 -> [w840]
                            tunnel: [w839] -> w793
                            tunnel: [w838] -> w794
                            tunnel: w798 -> [w847]
                            tunnel: w797 -> [w846]
                            frame #0 {
                              n153 = case shown="0, Default" w799 {
                                tunnel: [w807 w815 w823 w825 w829 w833] -> w800
                                frame 0, Default {
                                n154 = local read "RAM"() -> (w801:bool)
                                n155 = Number To Hexadecimal String(1:i16 4 ("width (-)"), 2:"P (PB1) Sollwert") -> (0:w808:string)
                                n156 = Select(t="*P17", s=w801, f="*W17") -> (s? t:f=w802:string)
                                n157 = Concatenate Strings(w802, w808) -> (w807:string)
                                }
                                frame 1 {
                                n158 = local read "RAM"() -> (w809:bool)
                                n159 = Number To Hexadecimal String(1:i16 4 ("width (-)"), 2:"I ( Reset1) Sollwert") -> (0:w816:string)
                                n160 = Select(t="*P18", s=w809, f="*W18") -> (s? t:f=w811:string)
                                n161 = Concatenate Strings(w811, w816) -> (w815:string)
                                }
                                frame 2 {
                                n162 = local read "RAM"() -> (w818:bool)
                                n163 = Number To Hexadecimal String(1:i16 4 ("width (-)"), 2:"D (Rate) Sollwert") -> (0:w824:string)
                                n164 = Select(t="*P19", s=w818, f="*W19") -> (s? t:f=w819:string)
                                n165 = Concatenate Strings(w819, w824) -> (w823:string)
                                }
                                frame 3 {
                                n166 = local read "RAM"() -> (w828:bool)
                                n167 = Select(t="*G17", s=w828, f="*R17") -> (s? t:f=w825:string)
                                }
                                frame 4 {
                                n168 = local read "RAM"() -> (w832:bool)
                                n169 = Select(t="*G18", s=w832, f="*R18") -> (s? t:f=w829:string)
                                }
                                frame 5 {
                                n170 = local read "RAM"() -> (w836:bool)
                                n171 = Select(t="*G19", s=w836, f="*R19") -> (s? t:f=w833:string)
                                }
                              }
                            }
                            frame #1 {
                              n172 = Unbundle(w840) -> ("VISA resource name out"=w845:refnum<visa-resource-name>, "error out"=w843:errorcluster, "Delay (ms)"=w844:u32, "Write/\nRead"=w842:bool)
                              n173 = call "I3252_Comm_Interface.vi"("VISA resource name in"=w845, "error in"=w843, "Delay (ms)"=w844, "Write"=w842, "String to Write"=w841, "Read"=w842) -> ("VISA resource name out"=w838:refnum<visa-resource-name>, "error out"=w839:errorcluster, "Read String"=w837:string)  [unwired: 2 in]
                            }
                            frame #2 {
                              n174 = case shown="5" w846 {
                                tunnel: w847 -> [_ w851 w855 w859]
                                frame 0, Default {
                                }
                                frame 3 {
                                n175 = String Subset(string=w851, offset (0)=3) -> (substring=w849:string)  [unwired: 1 in]
                                n176 = Hexadecimal String To Number(string=w849) -> (number=→"P (PB1) Istwert":u32)  [unwired: 2 in, 1 out]
                                }
                                frame 4 {
                                n177 = String Subset(string=w855, offset (0)=3) -> (substring=w853:string)  [unwired: 1 in]
                                n178 = Hexadecimal String To Number(string=w853) -> (number=→"I ( Reset1) Istwert":u32)  [unwired: 2 in, 1 out]
                                }
                                frame 5 {
                                n179 = String Subset(string=w859, offset (0)=3) -> (substring=w857:string)  [unwired: 1 in]
                                n180 = Hexadecimal String To Number(string=w857) -> (number=→"D (Rate) IstWert":u32)  [unwired: 2 in, 1 out]
                                }
                              }
                            }
                          }
                        }
                      }
                      frame #2 {
                        n181 = property on="Set PID" class="Bool"("Blinking"=FALSE) -> ()  [unwired: 2 in, 2 out]
                      }
                    }
                    n182 = Not(x="Set PID") -> (.not. x?=w786:bool)
                  }
                  event "Get Values": Value Change {
                    n183 = event-data() -> ()  [unwired: 1 in, 1 out]
                    n184 = stacked-sequence {
                      tunnel: w864 -> [_ w871 _]
                      tunnel: [_ w870 _] -> w863
                      tunnel: [_ w869 _] -> w862
                      frame #0 {
                        n185 = property on="Get Values" class="Bool"("Blinking"=TRUE) -> ()  [unwired: 2 in, 2 out]
                        n186 = property on="ON" class="Bool (strict)"("Blinking"=FALSE) -> ()  [unwired: 2 in, 2 out]
                      }
                      frame #1 {
                        n187 = for {
                          N: 6 -> [_]
                          tunnel: w871 -> [w875]
                          tunnel: [w874] -> w870
                          tunnel: [w873] -> w869
                          i -> [w877]
                          n188 = flat-sequence {
                            tunnel: w877 -> [w879]
                            tunnel: [w880] -> w876
                            tunnel: w876 -> [w902]
                            tunnel: [w903] -> w878
                            tunnel: w875 -> [w901]
                            tunnel: [w900] -> w873
                            tunnel: [w899] -> w874
                            tunnel: w878 -> [w909]
                            tunnel: w877 -> [w908]
                            frame #0 {
                              n189 = case shown="0, Default" w879 {
                                tunnel: [w883 w887 w891 "*R27" "*R28" w897] -> w880
                                frame 0, Default {
                                n190 = local read "RAM"() -> (w884:bool)
                                n191 = Select(t="*G17", s=w884, f="*R17") -> (s? t:f=w883:string)
                                }
                                frame 1 {
                                n192 = local read "RAM"() -> (w888:bool)
                                n193 = Select(t="*G18", s=w888, f="*R18") -> (s? t:f=w887:string)
                                }
                                frame 2 {
                                n194 = local read "RAM"() -> (w892:bool)
                                n195 = Select(t="*G19", s=w892, f="*R19") -> (s? t:f=w891:string)
                                }
                                frame 3 {
                                }
                                frame 4 {
                                }
                                frame 5 {
                                n196 = local read "RAM"() -> (w898:bool)
                                n197 = Select(t="*G01", s=w898, f="*R01") -> (s? t:f=w897:string)
                                }
                              }
                            }
                            frame #1 {
                              n198 = Unbundle(w901) -> ("VISA resource name out"=w907:refnum<visa-resource-name>, "error out"=w905:errorcluster, "Delay (ms)"=w906:u32, "Write/\nRead"=w904:bool)
                              n199 = call "I3252_Comm_Interface.vi"("VISA resource name in"=w907, "error in"=w905, "Delay (ms)"=w906, "Write"=w904, "String to Write"=w902, "Read"=w904) -> ("VISA resource name out"=w899:refnum<visa-resource-name>, "error out"=w900:errorcluster, "Read String"=w903:string)  [unwired: 2 in]
                            }
                            frame #2 {
                              n200 = case shown="0, Default" w908 {
                                tunnel: w909 -> [w911 w915 w919 w923 w927 w931]
                                frame 0, Default {
                                n201 = String Subset(string=w911, offset (0)=3) -> (substring=w912:string)  [unwired: 1 in]
                                n202 = Hexadecimal String To Number(string=w912) -> (number=w910:u32)  [unwired: 2 in, 1 out]
                                n203 = local write "P (PB1) Sollwert"(w910) -> ()
                                n204 = local write "P (PB1) Istwert"(w910) -> ()
                                }
                                frame 1 {
                                n205 = String Subset(string=w915, offset (0)=3) -> (substring=w916:string)  [unwired: 1 in]
                                n206 = Hexadecimal String To Number(string=w916) -> (number=w914:u32)  [unwired: 2 in, 1 out]
                                n207 = local write "I ( Reset1) Sollwert"(w914) -> ()
                                n208 = local write "I ( Reset1) Istwert"(w914) -> ()
                                }
                                frame 2 {
                                n209 = String Subset(string=w919, offset (0)=3) -> (substring=w920:string)  [unwired: 1 in]
                                n210 = Hexadecimal String To Number(string=w920) -> (number=w918:u32)  [unwired: 2 in, 1 out]
                                n211 = local write "D (Rate) Sollwert"(w918) -> ()
                                n212 = local write "D (Rate) IstWert"(w918) -> ()
                                }
                                frame 3 {
                                n213 = String Subset(string=w923, offset (0)=3) -> (substring=w924:string)  [unwired: 1 in]
                                n214 = Hexadecimal String To Number(string=w924) -> (number=w922:u32)  [unwired: 2 in, 1 out]
                                n215 = local write "% LOW Istwert"(w922) -> ()
                                n216 = local write "% LOW Sollwert"(w922) -> ()
                                }
                                frame 4 {
                                n217 = String Subset(string=w927, offset (0)=3) -> (substring=w928:string)  [unwired: 1 in]
                                n218 = Hexadecimal String To Number(string=w928) -> (number=w926:u32)  [unwired: 2 in, 1 out]
                                n219 = local write "% High Sollwert"(w926) -> ()
                                n220 = local write "% HIGH Istwert"(w926) -> ()
                                }
                                frame 5 {
                                n221 = call "I3252_Edit_Setpoint.vi"("Read String"=w931) -> ("Setpoint is"=w930:dbl)
                                n222 = local write "SP 1 is (°C)"(w930) -> ()
                                }
                              }
                            }
                          }
                        }
                      }
                      frame #2 {
                        n223 = property on="Get Values" class="Bool"("Blinking"=FALSE) -> ()  [unwired: 2 in, 2 out]
                      }
                    }
                    n224 = Not(x="Get Values") -> (.not. x?=w866:bool)
                  }
                  event "RAM": Value Change {
                    n225 = event-data() -> ()  [unwired: 1 in, 1 out]
                    n226 = stacked-sequence {
                      tunnel: w936 -> [_ w943 _]
                      tunnel: [_ w942 _] -> w935
                      tunnel: [_ w941 _] -> w934
                      frame #0 {
                        n227 = property on="RAM" class="Bool (strict)"("Blinking"=TRUE) -> ()  [unwired: 2 in, 2 out]
                        n228 = property on="ON" class="Bool (strict)"("Blinking"=FALSE) -> ()  [unwired: 2 in, 2 out]
                      }
                      frame #1 {
                        n229 = for {
                          N: 6 -> [_]
                          tunnel: w943 -> [w947]
                          tunnel: [w946] -> w942
                          tunnel: [w945] -> w941
                          i -> [w949]
                          n230 = flat-sequence {
                            tunnel: w949 -> [w951]
                            tunnel: [w952] -> w948
                            tunnel: w948 -> [w971]
                            tunnel: [w972] -> w950
                            tunnel: w947 -> [w975]
                            tunnel: [w974] -> w945
                            tunnel: [w973] -> w946
                            tunnel: w950 -> [w981]
                            tunnel: w949 -> [w980]
                            frame #0 {
                              n231 = case shown="0, Default" w951 {
                                tunnel: [w955 w959 w963 "*R27" "*R28" w969] -> w952
                                frame 0, Default {
                                n232 = local read "RAM"() -> (w956:bool)
                                n233 = Select(t="*G17", s=w956, f="*R17") -> (s? t:f=w955:string)
                                }
                                frame 1 {
                                n234 = local read "RAM"() -> (w960:bool)
                                n235 = Select(t="*G18", s=w960, f="*R18") -> (s? t:f=w959:string)
                                }
                                frame 2 {
                                n236 = local read "RAM"() -> (w964:bool)
                                n237 = Select(t="*G19", s=w964, f="*R19") -> (s? t:f=w963:string)
                                }
                                frame 3 {
                                }
                                frame 4 {
                                }
                                frame 5 {
                                n238 = local read "RAM"() -> (w970:bool)
                                n239 = Select(t="*G01", s=w970, f="*R01") -> (s? t:f=w969:string)
                                }
                              }
                            }
                            frame #1 {
                              n240 = Unbundle(w975) -> ("VISA resource name out"=w979:refnum<visa-resource-name>, "error out"=w977:errorcluster, "Delay (ms)"=w978:u32, "Write/\nRead"=w976:bool)
                              n241 = call "I3252_Comm_Interface.vi"("VISA resource name in"=w979, "error in"=w977, "Delay (ms)"=w978, "Write"=w976, "String to Write"=w971, "Read"=w976) -> ("VISA resource name out"=w973:refnum<visa-resource-name>, "error out"=w974:errorcluster, "Read String"=w972:string)  [unwired: 2 in]
                            }
                            frame #2 {
                              n242 = case shown="0, Default" w980 {
                                tunnel: w981 -> [w983 w987 w991 w995 w999 w1003]
                                frame 0, Default {
                                n243 = String Subset(string=w983, offset (0)=3) -> (substring=w984:string)  [unwired: 1 in]
                                n244 = Hexadecimal String To Number(string=w984) -> (number=w982:u32)  [unwired: 2 in, 1 out]
                                n245 = local write "P (PB1) Sollwert"(w982) -> ()
                                n246 = local write "P (PB1) Istwert"(w982) -> ()
                                }
                                frame 1 {
                                n247 = String Subset(string=w987, offset (0)=3) -> (substring=w988:string)  [unwired: 1 in]
                                n248 = Hexadecimal String To Number(string=w988) -> (number=w986:u32)  [unwired: 2 in, 1 out]
                                n249 = local write "I ( Reset1) Sollwert"(w986) -> ()
                                n250 = local write "I ( Reset1) Istwert"(w986) -> ()
                                }
                                frame 2 {
                                n251 = String Subset(string=w991, offset (0)=3) -> (substring=w992:string)  [unwired: 1 in]
                                n252 = Hexadecimal String To Number(string=w992) -> (number=w990:u32)  [unwired: 2 in, 1 out]
                                n253 = local write "D (Rate) IstWert"(w990) -> ()
                                n254 = local write "D (Rate) Sollwert"(w990) -> ()
                                }
                                frame 3 {
                                n255 = String Subset(string=w995, offset (0)=3) -> (substring=w996:string)  [unwired: 1 in]
                                n256 = Hexadecimal String To Number(string=w996) -> (number=w994:u32)  [unwired: 2 in, 1 out]
                                n257 = local write "% LOW Istwert"(w994) -> ()
                                n258 = local write "% LOW Sollwert"(w994) -> ()
                                }
                                frame 4 {
                                n259 = String Subset(string=w999, offset (0)=3) -> (substring=w1000:string)  [unwired: 1 in]
                                n260 = Hexadecimal String To Number(string=w1000) -> (number=w998:u32)  [unwired: 2 in, 1 out]
                                n261 = local write "% HIGH Istwert"(w998) -> ()
                                n262 = local write "% High Sollwert"(w998) -> ()
                                }
                                frame 5 {
                                n263 = call "I3252_Edit_Setpoint.vi"("Read String"=w1003) -> ("Setpoint is"=w1002:dbl)
                                n264 = local write "SP 1 is (°C)"(w1002) -> ()
                                }
                              }
                            }
                          }
                        }
                      }
                      frame #2 {
                        n265 = property on="RAM" class="Bool (strict)"("Blinking"=FALSE) -> ()  [unwired: 2 in, 2 out]
                      }
                    }
                    n266 = Not(x="RAM") -> (.not. x?=w938:bool)
                  }
                  event "Set Gauge to Zero": Value Change {
                    n267 = event-data() -> ()  [unwired: 1 in, 1 out]
                    n268 = flat-sequence {
                      tunnel: w1010 -> [w1015]
                      tunnel: [w1015] -> w1009
                      tunnel: w1009 -> [w1017]
                      tunnel: [w1021] -> w1008
                      tunnel: [w1020] -> w1007
                      tunnel: [w1017] -> w1006
                      tunnel: w1008 -> [w1027]
                      tunnel: w1007 -> [w1026]
                      tunnel: w1006 -> [w1022]
                      frame #0 {
                        n269 = property on="Set Gauge to Zero" class="Bool"("Blinking"=TRUE) -> ()  [unwired: 2 in, 2 out]
                      }
                      frame #1 {
                        w1018 = 0 items=["sensor 1", "sensor 2", "test"] ("Sensor Nr.:")
                        n270 = call "DUAL GAUGE-Get Pressure,Status.vi"("Sensor Nr.:"=w1018, "Referenz in"=w1017) -> ("Pressure"=w1021:dbl)  [unwired: 6 in, 3 out]
                        n271 = call "DUAL GAUGE-Offset display.vi"("W/R"=FALSE, "Referenz in"=w1017) -> ("Sensor 1 Get"=w1020:dbl)  [unwired: 6 in, 3 out]
                      }
                      frame #2 {
                        n272 = Add(x=w1027, y=w1026) -> (x+y=w1023:dbl)
                        n273 = call "DUAL GAUGE-Offset display.vi"("W/R"=TRUE, "Sensor 1 Set"=w1023, "Referenz in"=w1022) -> ("Sensor 1 Get"=→"Current Offset (mbar)":dbl)  [unwired: 5 in, 3 out]
                      }
                      frame #3 {
                        n274 = property on="Set Gauge to Zero" class="Bool"("Blinking"=TRUE) -> ()  [unwired: 2 in, 2 out]
                      }
                    }
                    n275 = Unbundle(w1014) -> ("VISA resource name out"=w1013:refnum<visa-resource-name>, "error out"=w1012:errorcluster)  [unwired: 2 out]
                  }
                  event "RAMP": Value Change {
                    n276 = event-data() -> ()  [unwired: 1 in, 4 out]
                    n277 = stacked-sequence {
                      tunnel: [_ w1038 _ _] -> w1030
                      tunnel: [_ w1037 _ _] -> w1031
                      tunnel: w1032 -> [_ w1036 w1094 _]
                      frame #0 {
                        n278 = property on="RAMP" class="Bool (strict)"("Blinking"=TRUE) -> ()  [unwired: 2 in, 2 out]
                      }
                      frame #1 {
                        n279 = for {
                          N: 6 -> [_]
                          tunnel: [w1044] -> w1038
                          tunnel: [w1043] -> w1037
                          tunnel: w1036 -> [w1042]
                          i -> [w1040]
                          n280 = flat-sequence {
                            tunnel: w1040 -> [w1046]
                            tunnel: [w1045] -> w1041
                            tunnel: [w1087] -> w1044
                            tunnel: [w1088] -> w1043
                            tunnel: w1042 -> [w1089]
                            tunnel: w1041 -> [w1086]
                            frame #0 {
                              n281 = case shown="2" w1046 {
                                tunnel: ["*D03" w1058 w1060 w1072 "*E03" ("string") "*Z02" ("string")] -> w1045
                                frame 0, Default {
                                }
                                frame 1 {
                                n282 = local read "RAMP"() -> (w1056:bool)
                                n283 = Select(t="*W0D78", s=w1056, f="*W0D60") -> (s? t:f=w1058:string)
                                n284 = Quotient & Remainder(x="Ramp time (min)", y=60.0) -> (x-y*floor(x/y)=w1055:dbl, floor(x/y)=w1054:dbl)
                                n285 = property on="Hours" class="DigNum (strict)"("Value"=w1054) -> ()  [unwired: 2 in, 2 out]
                                n286 = property on="Minutes" class="DigNum (strict)"("Value"=w1055) -> ()  [unwired: 2 in, 2 out]
                                n287 = Quotient & Remainder(x="Soak time (min)", y=60.0) -> (x-y*floor(x/y)=w1051:dbl, floor(x/y)=w1052:dbl)
                                n288 = property on="Soak Hours" class="DigNum (strict)"("Value"=w1052) -> ()  [unwired: 2 in, 2 out]
                                n289 = property on="Soak Minutes" class="DigNum (strict)"("Value"=w1051) -> ()  [unwired: 2 in, 2 out]
                                }
                                frame 2 {
                                n290 = local read "RAMP"() -> (w1061:bool)
                                n291 = case shown="True" w1061 {
                                tunnel: ["*W0E0000" ("string") w1063] -> w1060
                                frame False {
                                }
                                frame True {
                                n292 = Multiply(x="Hours", y=100.0) -> (x*y=w1069:dbl)
                                n293 = Add(x=w1069, y="Minutes") -> (x+y=w1066:dbl)
                                n294 = Number To Hexadecimal String(1:i16 4 ("width (-)"), 2:w1066) -> (0:w1067:string)
                                n295 = Concatenate Strings("*W0E" ("string"), w1067) -> (w1063:string)
                                }
                                }
                                }
                                frame 3 {
                                n296 = local read "RAMP"() -> (w1073:bool)
                                n297 = case shown="True" w1073 {
                                tunnel: ["*W1E0000" ("string") w1075] -> w1072
                                frame False {
                                }
                                frame True {
                                n298 = Multiply(x="Soak Hours", y=100.0) -> (x*y=w1081:dbl)
                                n299 = Add(x=w1081, y="Soak Minutes") -> (x+y=w1078:dbl)
                                n300 = Number To Hexadecimal String(1:i16 4 ("width (-)"), 2:w1078) -> (0:w1079:string)
                                n301 = Concatenate Strings("*W1E" ("string"), w1079) -> (w1075:string)
                                }
                                }
                                }
                                frame 4 {
                                }
                                frame 5 {
                                }
                              }
                            }
                            frame #1 {
                              n302 = Unbundle(w1089) -> ("VISA resource name out"=w1090:refnum<visa-resource-name>, "error out"=w1092:errorcluster, "Delay (ms)"=w1091:u32, "Write/\nRead"=w1093:bool)
                              n303 = call "I3252_Comm_Interface.vi"("VISA resource name in"=w1090, "error in"=w1092, "Delay (ms)"=w1091, "Write"=w1093, "String to Write"=w1086, "Read"=w1093) -> ("VISA resource name out"=w1088:refnum<visa-resource-name>, "error out"=w1087:errorcluster)  [unwired: 2 in, 1 out]
                            }
                          }
                          n304 = Wait (ms)(milliseconds to wait=u32 1000) -> ()  [unwired: 1 out]
                        }
                      }
                      frame #2 {
                        n305 = local read "RAMP"() -> (w1095:bool)
                        n306 = case shown="True" w1095 {
                          tunnel: w1094 -> [_ w1099]
                          frame False {
                          }
                          frame True {
                            n307 = property on="SP 1 input (°C)" class="DigNum (strict)"() -> ("Value"=w1098:dbl)  [unwired: 2 in, 2 out]
                            n308 = Multiply(x=10.0, y=w1098) -> (x*y=w1103:dbl)
                            n309 = Number To Hexadecimal String(1:i16 5 ("width (-)"), 2:w1103) -> (0:w1104:string)
                            n310 = Concatenate Strings("*P012", w1104) -> (w1101:string)
                            n311 = Wait (ms)(milliseconds to wait=u32 4000) -> ()  [unwired: 1 out]
                            n312 = Unbundle(w1099) -> ("VISA resource name out"=w1106:refnum<visa-resource-name>, "error out"=w1108:errorcluster, "Delay (ms)"=w1107:u32, "Write/\nRead"=w1109:bool)
                            n313 = call "I3252_Comm_Interface.vi"("VISA resource name in"=w1106, "error in"=w1108, "Delay (ms)"=w1107, "Write"=w1109, "String to Write"=w1101, "Read"=w1109) -> ("Read String"=w1096:string)  [unwired: 2 in, 2 out]
                            n314 = call "I3252_Edit_Setpoint.vi"("Read String"=w1096) -> ("Setpoint is"=w1097:dbl)
                            n315 = local write "SP 1 is (°C)"(w1097) -> ()
                          }
                        }
                      }
                      frame #3 {
                        n316 = property on="RAMP" class="Bool (strict)"("Blinking"=FALSE) -> ()  [unwired: 2 in, 2 out]
                      }
                    }
                    n317 = local read "RAMP"() -> (w1029:bool)
                  }
                  event "Get SetPoint": Value Change {
                    n318 = event-data() -> ()  [unwired: 1 in, 4 out]
                    n319 = Unbundle(w1118) -> ("VISA resource name out"=w1119:refnum<visa-resource-name>, "error out"=w1121:errorcluster, "Delay (ms)"=w1120:u32, "Write/\nRead"=w1122:bool)
                    n320 = call "I3252_Comm_Interface.vi"("VISA resource name in"=w1119, "error in"=w1121, "Delay (ms)"=w1120, "Write"=w1122, "String to Write"="*G01", "Read"=w1122) -> ("VISA resource name out"=w1116:refnum<visa-resource-name>, "error out"=w1114:errorcluster, "Read String"=w1117:string)  [unwired: 2 in]
                    n321 = call "I3252_Edit_Setpoint.vi"("Read String"=w1117) -> ("Setpoint is"=→"Actual SetPoint":dbl)
                  }
                  event "Write to File": Value Change {
                    n322 = event-data() -> ("NewVal"=w1129:bool)  [unwired: 1 in]
                    n323 = Unbundle(w1132) -> ("VISA resource name out"=w1131:refnum<visa-resource-name>, "error out"=w1130:errorcluster)  [unwired: 2 out]
                    n324 = local read "File Path"() -> (w1125:path)
                    n325 = case shown="True" w1129 {
                      tunnel: w1125 -> [_ w1137]
                      tunnel: "User" -> [_ w1136]
                      tunnel: "Sample" -> [_ w1135]
                      tunnel: [path "" ("File Path") w1134] -> w1126
                      frame False {
                      }
                      frame True {
                        n326 = call "Header.vi"("Sample"=w1135, "User"=w1136, "File Path"=w1137) -> ("File Path"=w1134:path)
                      }
                    }
                    n327 = local write "File Path"(w1126) -> ()
                  }
                }
              }
              n328 = Bundle(cluster=w444, "VISA resource name out"=w443, "error out"=w442) -> (w441:T7)  [unwired: 2 in]
            }
            frame #2 {
            }
            frame #3 {
              (unwired) "Daniel Schuster (geb. 20.03.1988)"
              n329 = property on="OUTPUT" class="Bool (strict)"() -> ("Value"=w1163:bool)  [unwired: 2 in, 2 out]
              n330 = node-c288(w1202) -> (w1211:T3)  [unwired: 2 in]
              n331 = node-c288(w1217) -> (w1220:T3)  [unwired: 2 in]
              n332 = node-c288(w1207) -> (w1209:T3)  [unwired: 2 in]
              n333 = node-c288(w1216) -> (w1224:T3)  [unwired: 2 in]
              n334 = case shown="True" w1163 {
                tunnel: [0.0 w1231] -> w1169
                tunnel: [0.0 w1230] -> w1166
                tunnel: [0.0 w1229] -> w1165
                tunnel: w1164 -> [_ w1228]
                frame False {
                }
                frame True {
                  n335 = flat-sequence {
                    tunnel: [w1256] -> w1252
                    tunnel: w1251 -> [w1255]
                    frame #0 {
                      n336 = Wait (ms)(milliseconds to wait=u32 300) -> ()  [unwired: 1 out]
                    }
                    frame #1 {
                      n337 = property class="Instr"(reference=w1255) -> ("Bytes at Port"=w1256:u32)  [unwired: 1 in, 2 out]
                    }
                  }
                  n338 = VISA Write(VISA resource name=w1228, write buffer=":MEAS:VOLT?;") -> (VISA resource name out=w1251:refnum<visa-resource-name>)  [unwired: 1 in, 2 out]
                  n339 = VISA Read(VISA resource name=w1251, byte count=w1252) -> (read buffer=w1245:string)  [unwired: 1 in, 3 out]
                  "read buffer" <- w1245
                  n340 = String Subset(string=w1245, offset (0)=1) -> (substring=w1244:string)  [unwired: 1 in]
                  n341 = Match Pattern(string=w1244, regular expression=",", offset (0)=1) -> (before substring=w1242:string, after substring=w1246:string)  [unwired: 2 out]
                  "Voltage\n 2" <- w1242
                  n342 = Fract/Exp String To Number(use system decimal point (T)=FALSE, string=w1242, offset=0) -> (number=w1229:dbl)  [unwired: 1 in, 1 out]
                  n343 = Match Pattern(string=w1246, regular expression=",", offset (0)=1) -> (before substring=w1241:string)  [unwired: 3 out]
                  "Current \n3" <- w1241
                  n344 = Fract/Exp String To Number(use system decimal point (T)=FALSE, string=w1241, offset=0) -> (number=w1230:dbl)  [unwired: 1 in, 1 out]
                  n345 = Divide(x=w1229, y=w1230) -> (x/y=w1236:dbl)
                  n346 = Compound Arithmetic op=MULTIPLY(w1236, "Thickness", 4.523 ("value"), "4PP Const", 1e-07 ("value")) -> (w1231:dbl)
                  "Resistivity\n 2" <- w1231
                }
              }
              n347 = timed-sequence {
                timing: w1211 -> [_]
                timing-out: [_] -> w1210
                tunnel: w1186 -> [w1299]
                tunnel: w1185 -> [w1295]
                tunnel: [w1298] -> w1178
                tunnel: w1177 -> [w1297]
                tunnel: w1176 -> [w1296]
                tunnel: [w1294] -> w1175
                tunnel: [w1293] -> w1174
                tunnel: [w1292] -> w1172
                n348 = timed-flat-sequence {
                  tunnel: w1299 -> [w1308]
                  tunnel: [w1307] -> w1298
                  tunnel: w1297 -> [w1306]
                  tunnel: w1296 -> [w1305]
                  tunnel: w1295 -> [w1304]
                  tunnel: [w1302] -> w1294
                  tunnel: [w1301] -> w1293
                  tunnel: [w1300] -> w1292
                  n349 = node-c288() -> ()  [unwired: 1 in, 1 out]
                  n350 = case shown="False" "ON (TPG 2)" {
                    tunnel: w1304 -> [w1313 w1319]
                    tunnel: w1305 -> [w1312 w1318]
                    tunnel: [w1311 w1317] -> w1301
                    tunnel: [w1310 w1316] -> w1300
                    frame False {
                      w1314 = 0.0 ("Pressure")
                      n351 = property on="ON (TPG 2)" class="Bool (strict)"("Blinking"=FALSE) -> ()  [unwired: 2 in, 2 out]
                      n352 = Bundle("Pressure"=w1314, "Pressure"=w1314) -> (w1311:cluster{"Pressure":dbl, "Pressure":dbl})  [unwired: 1 in]
                      n353 = Bundle("TPG 2 COM"=w1313, "error out"=w1312) -> (w1310:T8)  [unwired: 1 in]
                    }
                    frame True {
                      n354 = stacked-sequence {
                        tunnel: w1319 -> [_ w1332]
                        tunnel: [_ w1328] -> w1317
                        tunnel: [_ w1324] -> w1316
                        tunnel: w1318 -> [_ w1321]
                        frame #0 {
                          n355 = property on="ON (TPG 2)" class="Bool (strict)"("Blinking"=TRUE) -> ()  [unwired: 2 in, 2 out]
                        }
                        frame #1 {
                          n356 = call "PresureGetSubVI.vi"("COM in"=w1332, "Fehler (Eingang)"=w1321) -> ("Status Gauge#1"=→"Status Gauge 2#1":i32, "Status Gauge#2"=→"Status Gauge 2#2":i32, "COM out"=w1325:refnum<visa-resource-name>, "Pressure Gauge#1"=w1326:dbl, "Pressure Gauge#2"=w1329:dbl, "Cluster (Ausgang)"=w1322:errorcluster)  [unwired: 12 in]
                          "Pressure Gauge 2#1" <- w1326
                          "Pressure Gauge 2#2" <- w1329
                          n357 = Bundle("COM out"=w1325, "Cluster (Ausgang)"=w1322) -> (w1324:T9)  [unwired: 1 in]
                          n358 = Unbundle(w1322) -> ("status"=w1323:bool, "code"=w1327:i32)  [unwired: 1 out]
                          n359 = Bundle("status"=w1323, "code"=w1327) -> ()  [unwired: 1 in, 1 out]
                          n360 = Bundle("Pressure Gauge#1"=w1326, "Pressure Gauge#2"=w1329) -> (w1328:T10)  [unwired: 1 in]
                        }
                      }
                    }
                  }
                  n361 = case shown="True" "ON (TPG 1)" {
                    tunnel: w1308 -> [w1336 w1342]
                    tunnel: [w1335 w1341] -> w1307
                    tunnel: w1306 -> [w1334 w1340]
                    tunnel: [w1333 w1339] -> w1302
                    frame False {
                      w1337 = 0.0 ("Pressure")
                      n362 = property on="ON (TPG 1)" class="Bool (strict)"("Blinking"=FALSE) -> ()  [unwired: 2 in, 2 out]
                      n363 = Bundle("Pressure"=w1337, "Pressure"=w1337) -> (w1333:cluster{"Pressure":dbl, "Pressure":dbl})  [unwired: 1 in]
                      n364 = Bundle("TPG 1 COM"=w1336, "error out"=w1334) -> (w1335:T11)  [unwired: 1 in]
                    }
                    frame True {
                      n365 = stacked-sequence {
                        tunnel: w1342 -> [_ w1355]
                        tunnel: [_ w1348] -> w1341
                        tunnel: w1340 -> [_ w1345]
                        tunnel: [_ w1344] -> w1339
                        frame #0 {
                          n366 = property on="ON (TPG 1)" class="Bool (strict)"("Blinking"=TRUE) -> ()  [unwired: 2 in, 2 out]
                        }
                        frame #1 {
                          n367 = call "PresureGetSubVI.vi"("COM in"=w1355, "Fehler (Eingang)"=w1345) -> ("Status Gauge#1"=→"Status Gauge 1#1":i32, "Status Gauge#2"=→"Status Gauge 1#2":i32, "COM out"=w1349:refnum<visa-resource-name>, "Pressure Gauge#1"=w1350:dbl, "Pressure Gauge#2"=w1352:dbl, "Cluster (Ausgang)"=w1346:errorcluster)  [unwired: 12 in]
                          "Pressure Gauge 1#1" <- w1350
                          "Pressure Gauge 1#2" <- w1352
                          n368 = Bundle("COM out"=w1349, "Cluster (Ausgang)"=w1346) -> (w1348:T9)  [unwired: 1 in]
                          n369 = Unbundle(w1346) -> ("status"=w1347:bool, "code"=w1351:i32)  [unwired: 1 out]
                          n370 = Bundle("status"=w1347, "code"=w1351) -> ()  [unwired: 1 in, 1 out]
                          n371 = Bundle("Pressure Gauge#1"=w1350, "Pressure Gauge#2"=w1352) -> (w1344:T10)  [unwired: 1 in]
                        }
                      }
                    }
                  }
                  n372 = node-c288() -> ()  [unwired: 1 in, 1 out]
                }
              }
              n373 = timed-sequence {
                timing: w1220 -> [_]
                timing-out: [_] -> w1219
                tunnel: w1218 -> [w1365]
                tunnel: [w1364] -> w1213
                tunnel: [w1363] -> w1212
                tunnel: [w1362] -> w1199
                n374 = timed-flat-sequence {
                  tunnel: w1365 -> [w1369]
                  tunnel: [w1368] -> w1364
                  tunnel: [w1367] -> w1363
                  tunnel: [w1366] -> w1362
                  n375 = node-c288() -> ()  [unwired: 1 in, 1 out]
                  n376 = case shown="True" "ON" {
                    tunnel: w1369 -> [w1373 w1378]
                    tunnel: [w1372 w1377] -> w1368
                    tunnel: [w1371 w1376] -> w1367
                    tunnel: [_ w1375] -> w1366
                    frame False {
                      n377 = Unbundle(w1373) -> ("VISA resource name out"=w1372:refnum<visa-resource-name>, "error out"=w1371:errorcluster)  [unwired: 2 out]
                      n378 = property on="ON" class="Bool (strict)"("Blinking"=FALSE) -> ()  [unwired: 2 in, 2 out]
                    }
                    frame True {
                      n379 = stacked-sequence {
                        tunnel: w1378 -> [_ w1383]
                        tunnel: [_ w1382] -> w1377
                        tunnel: [_ w1381] -> w1376
                        tunnel: [_ w1380] -> w1375
                        frame #0 {
                          n380 = property on="ON" class="Bool (strict)"("Blinking"=TRUE) -> ()  [unwired: 2 in, 2 out]
                        }
                        frame #1 {
                          n381 = Unbundle(w1383) -> ("VISA resource name out"=w1387:refnum<visa-resource-name>, "error out"=w1385:errorcluster, "Delay (ms)"=w1386:u32, "Write/\nRead"=w1384:bool)
                          n382 = call "I3252_Comm_Interface.vi"("VISA resource name in"=w1387, "error in"=w1385, "Delay (ms)"=w1386, "Write"=w1384, "String to Write"="*V01", "Read"=w1384) -> ("VISA resource name out"=w1382:refnum<visa-resource-name>, "error out"=w1381:errorcluster, "Read String"=w1380:string)  [unwired: 2 in]
                        }
                      }
                    }
                  }
                  n383 = node-c288() -> ()  [unwired: 1 in, 1 out]
                }
              }
              n384 = timed-sequence {
                timing: w1209 -> [_]
                timing-out: [_] -> w1208
                tunnel: w1206 -> [w1261]
                tunnel: w1205 -> [w1260]
                tunnel: [w1259] -> w1203
                tunnel: [w1258] -> w1204
                tunnel: [w1257] -> w1200
                n385 = timed-flat-sequence {
                  tunnel: w1261 -> [w1266]
                  tunnel: w1260 -> [w1265]
                  tunnel: [w1264] -> w1259
                  tunnel: [w1263] -> w1258
                  tunnel: [w1262] -> w1257
                  n386 = node-c288() -> ()  [unwired: 1 in, 1 out]
                  n387 = case shown="False" "ON" {
                    tunnel: w1266 -> [w1270 w1276]
                    tunnel: w1265 -> [w1271 w1275]
                    tunnel: [w1270 w1274] -> w1264
                    tunnel: [w1271 w1273] -> w1263
                    tunnel: [0.0 ("Reading") w1272] -> w1262
                    frame False {
                      n388 = property on="ON" class="Bool (strict)"("Blinking"=FALSE) -> ()  [unwired: 2 in, 2 out]
                    }
                    frame True {
                      n389 = stacked-sequence {
                        tunnel: w1276 -> [_ w1283]
                        tunnel: w1275 -> [_ w1282]
                        tunnel: [_ w1281] -> w1274
                        tunnel: [_ w1280] -> w1273
                        tunnel: [_ w1278] -> w1272
                        frame #0 {
                          n390 = property on="ON" class="Bool (strict)"("Blinking"=TRUE) -> ()  [unwired: 2 in, 2 out]
                        }
                        frame #1 {
                          n391 = call "VC840_Read.vi"("error in (no error)"=w1282, "VISA resource name"=w1283) -> ("error out"=w1280:errorcluster, "Unit"=→"Unit 2":string, "Reading"=w1278:dbl, "VISA resource name out"=w1281:refnum<visa-resource-name>, "Status"=→"Status 2":T2, "Mode"=→"Mode 2":enum16{"?", "Diode", "Beep", "DC", "AC"})  [unwired: 4 out]
                          "Reading 2" <- w1278
                        }
                      }
                    }
                  }
                  n392 = node-c288() -> ()  [unwired: 1 in, 1 out]
                }
              }
              n393 = timed-sequence {
                timing: w1224 -> [_]
                timing-out: [_] -> w1223
                tunnel: w1222 -> [w1399]
                tunnel: w1221 -> [w1398]
                tunnel: [w1397] -> w1215
                tunnel: [w1396] -> w1214
                tunnel: [w1395] -> w1201
                n394 = timed-flat-sequence {
                  tunnel: w1399 -> [w1404]
                  tunnel: w1398 -> [w1403]
                  tunnel: [w1402] -> w1397
                  tunnel: [w1401] -> w1396
                  tunnel: [w1400] -> w1395
                  n395 = node-c288() -> ()  [unwired: 1 in, 1 out]
                  n396 = case shown="False" "ON" {
                    tunnel: w1404 -> [w1408 w1414]
                    tunnel: w1403 -> [w1409 w1413]
                    tunnel: [w1408 w1412] -> w1402
                    tunnel: [w1409 w1411] -> w1401
                    tunnel: [0.0 ("Reading") w1410] -> w1400
                    frame False {
                      n397 = property on="ON" class="Bool (strict)"("Blinking"=FALSE) -> ()  [unwired: 2 in, 2 out]
                    }
                    frame True {
                      n398 = stacked-sequence {
                        tunnel: w1414 -> [_ w1421]
                        tunnel: w1413 -> [_ w1420]
                        tunnel: [_ w1419] -> w1412
                        tunnel: [_ w1418] -> w1411
                        tunnel: [_ w1416] -> w1410
                        frame #0 {
                          n399 = property on="ON" class="Bool (strict)"("Blinking"=TRUE) -> ()  [unwired: 2 in, 2 out]
                        }
                        frame #1 {
                          n400 = call "VC840_Read.vi"("error in (no error)"=w1420, "VISA resource name"=w1421) -> ("error out"=w1418:errorcluster, "Unit"=→"Unit 1":string, "Reading"=w1416:dbl, "VISA resource name out"=w1419:refnum<visa-resource-name>, "Status"=→"Status 1":T2, "Mode"=→"Mode 1":enum16{"?", "Diode", "Beep", "DC", "AC"})  [unwired: 4 out]
                          "Reading 1" <- w1416
                        }
                      }
                    }
                  }
                  n401 = node-c288() -> ()  [unwired: 1 in, 1 out]
                }
              }
              n402 = Tick Count (ms)() -> (millisecond timer value=w1187:u32)
              n403 = Subtract(x=w1187, y=w1192) -> (x-y=w1191:u32)
              n404 = Divide(x=w1191, y=u32 1000) -> (x/y=w1189:dbl)
              n405 = node-c288(w1223) -> ()  [unwired: 1 out]
              n406 = node-c288(w1208) -> ()  [unwired: 1 out]
              n407 = node-c288(w1219) -> ()  [unwired: 1 out]
              n408 = To Double Precision Float(number=w1189) -> (double precision float=w1193:dbl)
              "current time (s)" <- w1193
              n409 = node-c288(w1210) -> ()  [unwired: 1 out]
              n410 = Unbundle(w1174) -> ("Pressure Gauge#1"=w1173:dbl, "Pressure Gauge#2"=w1171:dbl)
              "Pressure Pirani 2" <- w1173
              n411 = Unbundle(w1175) -> ("Pressure Gauge#1"=w1184:dbl, "Pressure Gauge#2"=w1179:dbl)
              "Pressure Baratron 2" <- w1184
            }
            frame #4 {
              n412 = Build Array (concatenate)(w1451, w1455) -> (w1450:dbl[])
              n413 = Build Array (concatenate)(w1454, w1456) -> (w1449:dbl[])
              n414 = Build Array (concatenate)(w1452, w1443) -> (w1447:dbl[])
              n415 = Build Array (concatenate)(w1453, w1444) -> (w1448:dbl[])
              n416 = Build Array (concatenate)(w1439, w1431) -> (w1438:dbl[])
              n417 = Build Array (concatenate)(w1437, w1433) -> (w1434:dbl[])
              n418 = Build Array (concatenate)(w1436, w1432) -> (w1435:dbl[])
              n419 = Greater?(x=w1475, y="Pressure Limit (mbar)") -> (0:w1478:bool)
              n420 = case shown="False" w1478 {
                frame False {
                  n421 = property on="Standby" class="Bool (strict)"("DisabledEnum"=T6."Enabled" ("Disabled")) -> ()  [unwired: 2 in, 2 out]
                }
                frame True {
                  n422 = property on="Standby" class="Bool (strict)"("Val(Sgnl)"=TRUE ("Standby"), "DisabledEnum"=T6."Disabled" ("Disabled")) -> ()  [unwired: 2 in, 2 out]
                }
              }
              n423 = call "Resistivity_Calculation.vi"("Reading 1 (V)"=w1468, "Constant"="4PP constant", "Thickness (nm)"="Thickness (nm)", "Reading 2 (A)"=w1476) -> ("Resivtivity (Ohm*cm)"=w1460:dbl, "Current"=w1461:dbl, "Voltage"=w1462:dbl)
              n424 = call "I3252_Edit_Temperature.vi"("Temp. String"=w1477) -> ("Temp. (°C)"=w1471:dbl)
              "(°C)" <- w1471
              n425 = Build Array(w1432, w1433, w1431) -> (w1430:dbl[])
              n426 = Build Array (concatenate)(w1473, w1474) -> (w1470:dbl[])
              n427 = Build Array (concatenate)(w1472, w1471) -> (w1458:dbl[])
              n428 = Build Array (concatenate)(w1469, w1462) -> (w1467:dbl[])
              n429 = Build Array (concatenate)(w1466, w1461) -> (w1464:dbl[])
              n430 = Build Array (concatenate)(w1465, w1460) -> (w1463:dbl[])
              n431 = Build Array(w1462, w1461, w1460) -> (w1459:dbl[])
            }
            frame #5 {
              n432 = Bundle(w1499, w1498) -> (→"Voltage Graph":cluster{dbl[], dbl[]})  [unwired: 1 in]
              n433 = Bundle(w1491, w1492) -> (→"Resistivity/ Temp Dependency":cluster{dbl[], dbl[]})  [unwired: 1 in]
              n434 = Bundle(w1499, w1497) -> (→"Current Graph":cluster{dbl[], dbl[]})  [unwired: 1 in]
              n435 = Bundle(w1499, w1492) -> (→"Resistivity Graph":cluster{dbl[], dbl[]})  [unwired: 1 in]
              n436 = Bundle(w1499, w1513) -> (→"TPG 1":cluster{dbl[], dbl[]})  [unwired: 1 in]
              n437 = Bundle(w1499, w1512) -> ()  [unwired: 1 in, 1 out]
              n438 = Bundle(w1499, w1511) -> (→"Pirani (VVP1 Scroll)":cluster{dbl[], dbl[]})  [unwired: 1 in]
              n439 = Bundle(w1499, w1510) -> ()  [unwired: 1 in, 1 out]
              n440 = Bundle(w1499, w1491) -> (→"Thermocouple":cluster{dbl[], dbl[]})  [unwired: 1 in]
              n441 = Bundle(w1499, w1517) -> ()  [unwired: 1 in, 1 out]
              n442 = Bundle(w1499, w1518) -> ()  [unwired: 1 in, 1 out]
              n443 = Bundle(w1499, w1519) -> ()  [unwired: 1 in, 1 out]
              n444 = Build Array (concatenate)(w1515, w1520, w1495, w1494) -> (w1527:dbl[])
              "appended array" <- w1527
            }
            frame #6 {
              n445 = Unbundle(w1536) -> ("COM out"=w1535:refnum<visa-resource-name>, "Cluster (Ausgang)"=w1534:errorcluster)
              n446 = Unbundle(w1533) -> ("COM out"=w1532:refnum<visa-resource-name>, "Cluster (Ausgang)"=w1531:errorcluster)
              n447 = case shown="False" "Write to File" {
                tunnel: [_ w1564] -> w1550
                tunnel: "File Path" -> [_ w1562]
                tunnel: w1543 -> [_ w1560]
                frame False {
                  n448 = property on="Write to File" class="Bool (strict)"("Blinking"=FALSE) -> ()  [unwired: 2 in, 2 out]
                }
                frame True {
                  n449 = flat-sequence {
                    tunnel: [w1566] -> w1563
                    tunnel: w1562 -> [w1566]
                    tunnel: [w1565] -> w1561
                    tunnel: w1560 -> [w1565]
                    tunnel: [w1571] -> w1564
                    tunnel: w1563 -> [w1570]
                    tunnel: w1561 -> [w1569]
                    frame #0 {
                      n450 = property on="Write to File" class="Bool (strict)"("Blinking"=TRUE) -> ()  [unwired: 2 in, 2 out]
                    }
                    frame #1 {
                      n451 = call-poly <vilib>:"Write To Spreadsheet File.vi"("format (%.3f)"="%g", "append to file? (new file:F)"=TRUE ("transpose? (no:F)"), "1D data"=w1569, "file path (dialog if empty)"=w1570) -> ("new file path (Not A Path if cancelled)"=w1571:path)  [unwired: 4 in]
                    }
                  }
                }
              }
              n452 = Merge Errors(w1555, w1554, w1552, w1534, w1531) -> (w1553:errorcluster)
              n453 = call <vilib>:"Simple Error Handler.vi"("error in (no error)"=w1553) -> ("error?"=w1537:bool)  [unwired: 4 in, 4 out]
              n454 = local write "File Path"(w1550) -> ()
            }
            frame #7 {
              w1590 = u32 1000 ("y")
              n455 = Tick Count (ms)() -> (millisecond timer value=w1592:u32)
              n456 = Subtract(x=w1592, y=w1591) -> (x-y=w1593:u32)
              n457 = VISA Flush I/O Buffer(VISA resource name=w1584, error in (no error)=w1583) -> (VISA resource name out=w1581:refnum<visa-resource-name>, error out=w1582:errorcluster)  [unwired: 1 in]
              n458 = VISA Flush I/O Buffer(VISA resource name=w1577, error in (no error)=w1576) -> (VISA resource name out=w1580:refnum<visa-resource-name>, error out=w1579:errorcluster)  [unwired: 1 in]
              n459 = Divide(x=w1593, y=w1590) -> (x/y=→"loop time (s)":dbl)
              n460 = Subtract(x="Intervall (s)", y=u32 1) -> (x-y=w1594:u32)
              n461 = Multiply(x=w1594, y=w1590) -> (x*y=w1597:u32)
              n462 = Wait (ms)(milliseconds to wait=w1597) -> ()  [unwired: 1 out]
              n463 = Bundle("COM out"=w1581, "error out"=w1582, "COM out"=w1580, "error out"=w1579) -> (w1578:T12)  [unwired: 1 in]
            }
            frame #8 {
              n464 = Tick Count (ms)() -> (millisecond timer value=w1620:u32)
              n465 = Subtract(x=w1620, y=w1618) -> (x-y=w1619:u32)
              n466 = Divide(x=w1619, y=w1617) -> (x/y=→"data logger intervall (s)":dbl)
            }
          }
          n467 = Exclusive Or(1:"stop", 2:w198) -> (0:w199:bool)
        }
      }
      frame #4 {
        n468 = call "VC840_Close.vi"("error in (no error)"=w1639, "VISA resource name"=w1640) -> ("error out"=w1648:errorcluster)  [unwired: 9 in]
        n469 = call "VC840_Close.vi"("error in (no error)"=w1641, "VISA resource name"=w1642) -> ("error out"=w1646:errorcluster)  [unwired: 9 in]
        n470 = VISA Close(VISA resource name=w1644, error in (no error)=w1643) -> (error out=w1645:errorcluster)
        n471 = Unbundle(w1637) -> ("COM out"=w1636:refnum<visa-resource-name>, "error out"=w1635:errorcluster, "COM out"=w1633:refnum<visa-resource-name>, "error out"=w1634:errorcluster)
        n472 = VISA Close(VISA resource name=w1636, error in (no error)=w1635) -> ()  [unwired: 1 out]
        n473 = VISA Close(VISA resource name=w1633, error in (no error)=w1634) -> ()  [unwired: 1 out]
        n474 = Merge Errors(w1645, w1646, w1648) -> (w1647:errorcluster)
        n475 = call <vilib>:"Simple Error Handler.vi"("error in (no error)"=w1647) -> ("error?"=w1638:bool)  [unwired: 1 in, 7 out]
        n476 = Stop(stop? (T)=w1638) -> ()
      }
    }
  }
